vi "Main.vi"() -> ()   [LabVIEW 2020]
uses:
  <vilib>/MediaMongrels Ltd/WebSockets/Sockets/VISA TCP Listener/VISA TCP Listener.lvclass
  <vilib>/MediaMongrels Ltd/WebSockets/WebSockets/WebSocket Server/WebSocket Server.lvclass
  <vilib>/MediaMongrels Ltd/WebSockets/Sockets/Socket/Socket.lvclass
  <vilib>/Skyline/Tag/Wrapper/Wrapper_class/NI Skyline Tag.lvclass
  <vilib>/Skyline/Message/HTTP Wrapper/NI Skyline Message HTTP.lvclass
  <vilib>/Skyline/Tag/Shared/typedefs/DataType.ctl
  <vilib>/Skyline/Configuration/Configuration HTTP_class/NI Skyline Configuration HTTP.lvclass/NI Skyline Configuration HTTP.ctl
  <vilib>/Skyline/Configuration/Configuration HTTP_class/Open Configuration API Key.vi
  <vilib>/Skyline/Configuration/HTTP/Open Configuration API Key (Desktop).vi
  <vilib>/Skyline/Message/HTTP Wrapper/Open (HTTP).vi
  <vilib>/Skyline/Tag/Wrapper/Wrapper HTTP_class/Open Tag HTTP.vi
  <vilib>/Skyline/Tag/Wrapper/Wrapper_class/Write Tag (String).vi
  <vilib>/Skyline/Tag/Wrapper/Wrapper_class/Write Tag (Boolean).vi
  <vilib>/Skyline/Tag/Wrapper/Wrapper_class/Close Tag (Single).vi
  <vilib>/ErrorRing/Error Ring.xnode
  <vilib>/Skyline/Configuration/Configuration HTTP_class/NI Skyline Configuration HTTP.lvclass
  <vilib>/addons/_JKI.lib/Serialization/JSON/JKI JSON Serialization.lvlib
  <vilib>/Skyline/Configuration/Configuration_class/NI Skyline Configuration.lvclass
  <vilib>/Skyline/Tag/Shared/NI Skyline Tag.lvlib
  <vilib>/Skyline/Tag/Wrapper/Wrapper HTTP_class/NI Skyline Tag HTTP.lvclass
  <vilib>/Skyline/Message/NI Skyline Message.lvclass
panel:
  in  "Send SystemLink Messages?":bool
  in  "Send SystemLink Tags?":bool
  in  "Sync":bool
  out "Pi OS Time":string
  out "LV OS Time":string
  in  "LV Enabled":bool
  in  "LV OS Enabled":bool
  in  "Pi OS Enabled":bool
  in  "Pi OS TZ Update":bool
  in  "LV OS TZ Update":bool
  in  "LV TZ Update":bool
  out "LV Time":string
  in  "Timezone":string(combo)
  in  "Stop":bool
  # "Raspberry Pi WebSocket Server Example"
  # "This simple example sends the current date/time to the connected WebSocket Client.\n\nTo be used in conjunction with the corresponding NXG WebVI."
  # "Timezone\nUpdate"
  # "Update\nEnabled"
  # "Last Time Received"
  # "LabVIEW"
  # "LabVIEW OS"
  # "Pi OS"
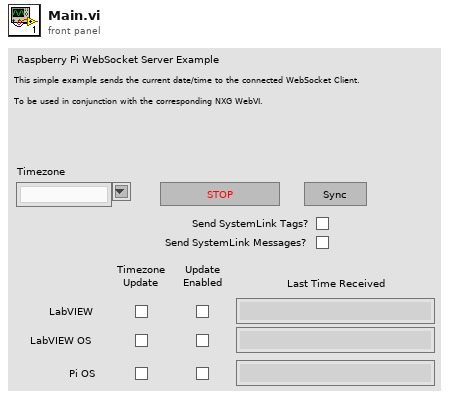
[diagram p1: front panel]
types:
  T1 = cluster{"Command":string, "Controls":cluster{"Name":string, "Value":bool}[]}
  T2 = typedef "NI Skyline Tag.lvlib/DataType.ctl" = enum32{"Double", "I32", "String", "Boolean", "U64", "Timestamp"}
  T3 = cluster{"Name":string, "Reference":refnum<class "NI Skyline Tag.lvclass">}
  T4 = cluster{"Core":cluster{"Current VI Reference":refnum<vi>}, "TCP Listener":refnum<class "VISA TCP Listener.lvclass">, "Socket":refnum<class "Socket.lvclass">, "WebSocket":refnum<class "WebSocket Server.lvclass">, "TCP Connection Info":cluster{"TCP Listen Port":u16, "Timeout (ms)":i32}, "Current Timezone":string, "Websocket Connected?":bool, "Current Time":cluster{"LabVIEW":string, "LabVIEW OS":string, "Pi OS":string}, "JSON Data In":string, "JSON Data Out":string, "Enabled Booleans":cluster{"LV Enabled":bool, "LV OS Enabled":bool, "Pi OS Enabled":bool}, "Timezone Booleans":cluster{"LV TZ Update":bool, "LV OS TZ Update":bool, "Pi OS TZ Update":bool}, "Initialized?":bool, "SystemLink Tag Info":cluster{"Name":string, "Reference":refnum<class "NI Skyline Tag.lvclass">}[], "SystemLink Booleans":cluster{"Send SystemLink Tags?":bool, "Send SystemLink Messages?":bool}, "SystemLink Message Session":refnum<class "NI Skyline Message HTTP.lvclass">}
  T5 = cluster{"Send SystemLink Tags?":bool, "Send SystemLink Messages?":bool}
  T6 = cluster{"Name":string, "Reference":refnum<class "NI Skyline Tag.lvclass">}[]
  T7 = cluster{"LV TZ Update":bool, "LV OS TZ Update":bool, "Pi OS TZ Update":bool}
  T8 = cluster{"LV Enabled":bool, "LV OS Enabled":bool, "Pi OS Enabled":bool}
  T9 = cluster{"LabVIEW":string, "LabVIEW OS":string, "Pi OS":string}
  T10 = cluster{"TCP Listen Port":u16, "Timeout (ms)":i32}
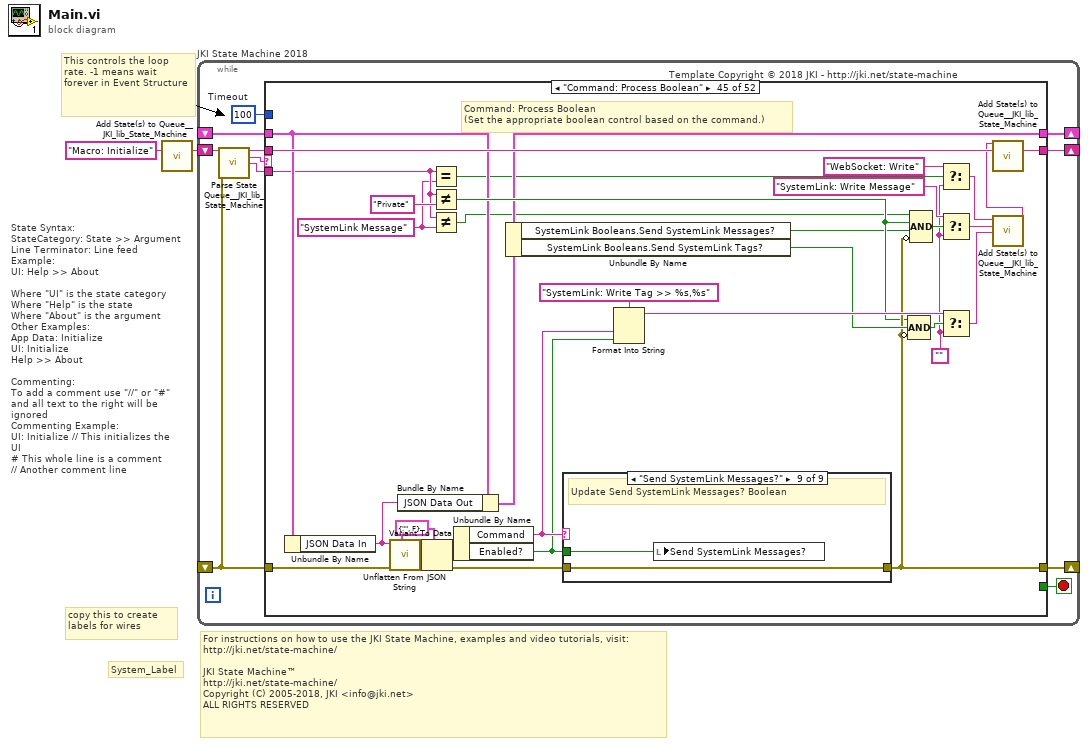
[diagram p0: block diagram]
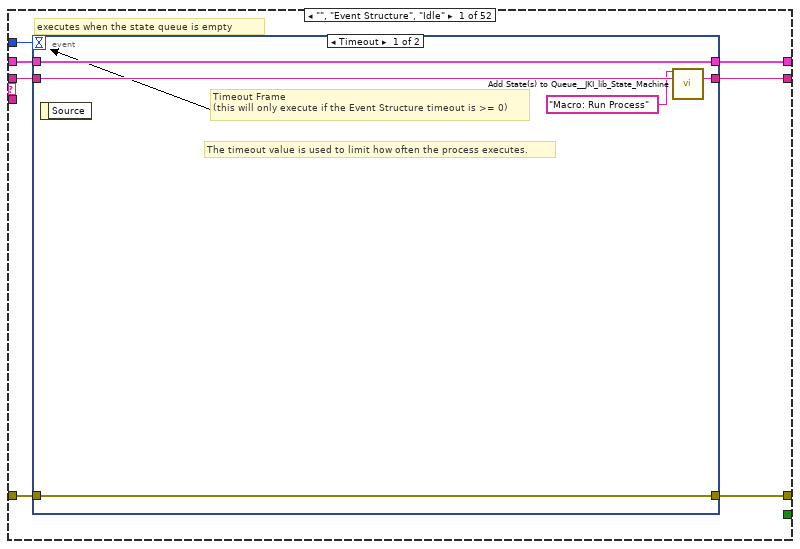
[diagram p2: hidden frame]
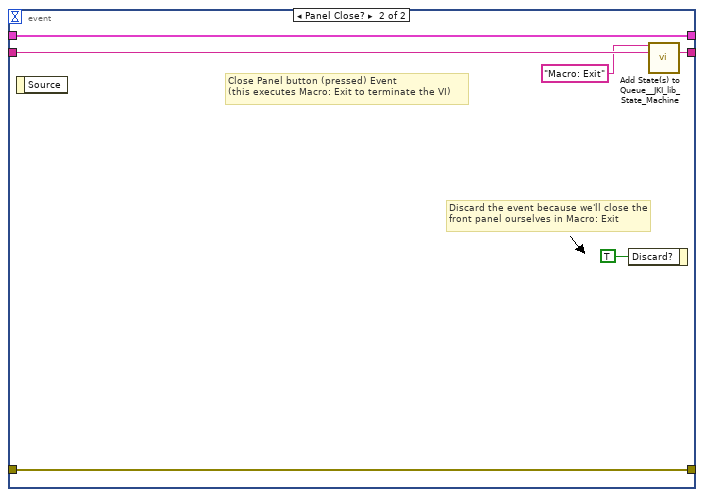
[diagram p3: hidden frame]
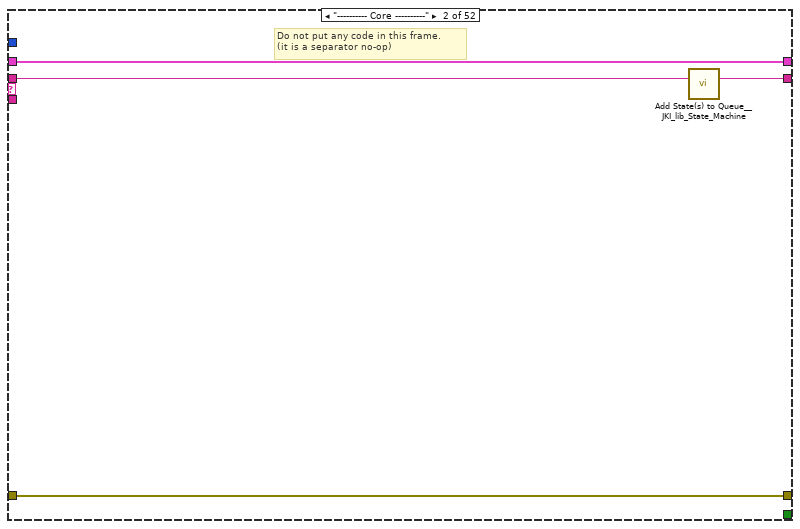
[diagram p4: hidden frame]
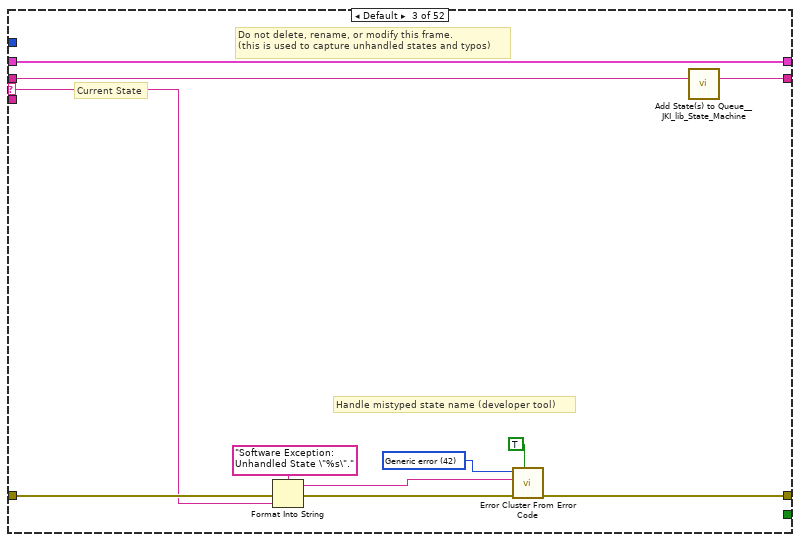
[diagram p5: hidden frame]
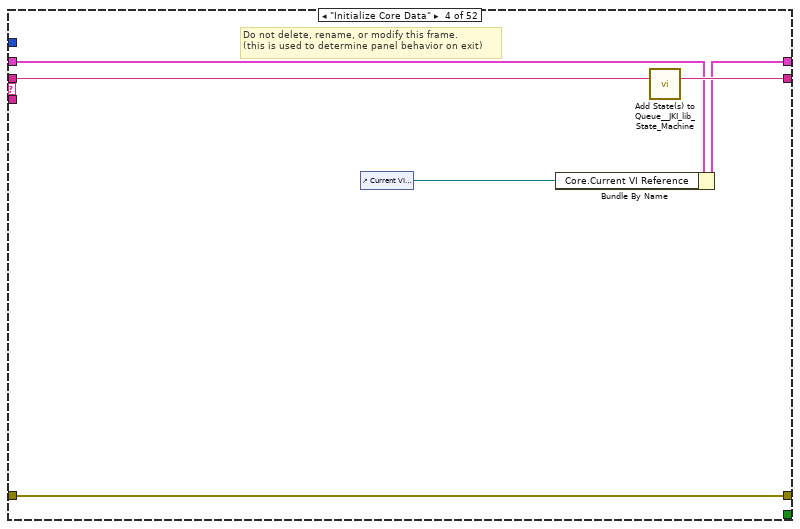
[diagram p6: hidden frame]
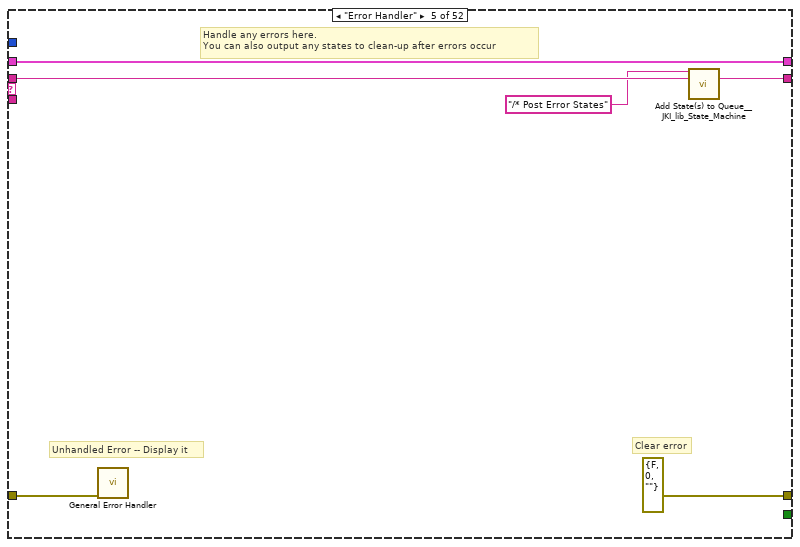
[diagram p7: hidden frame]
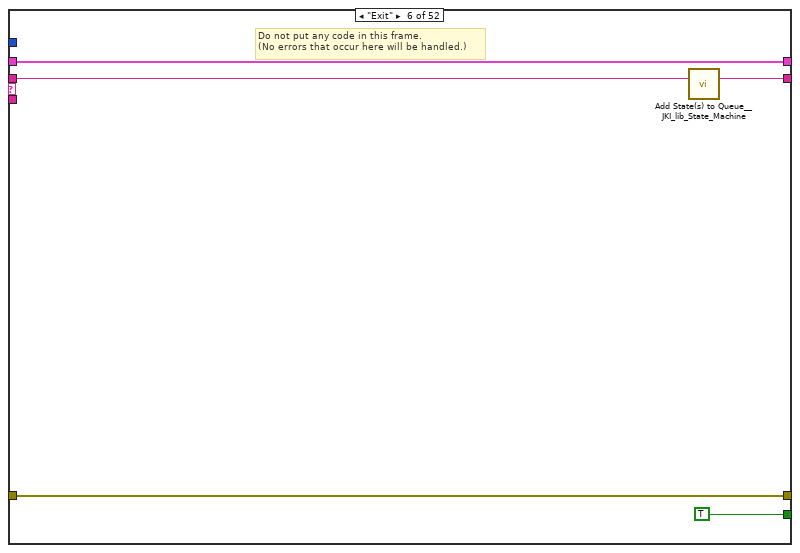
[diagram p8: hidden frame]
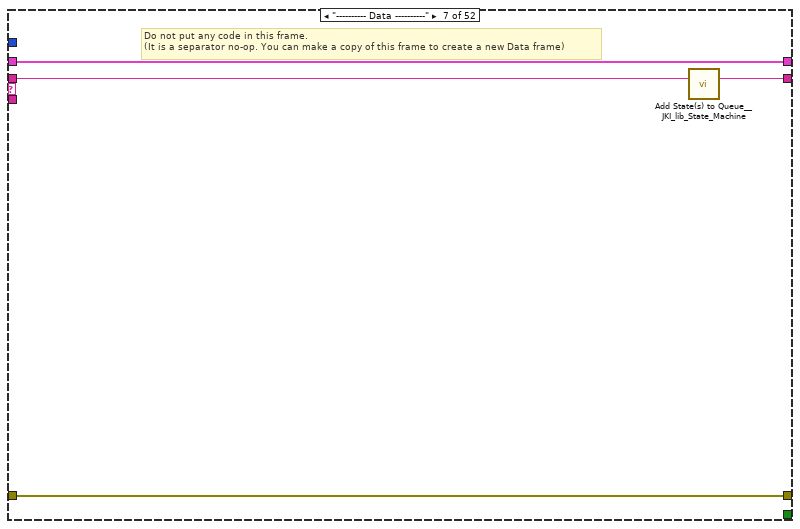
[diagram p9: hidden frame]
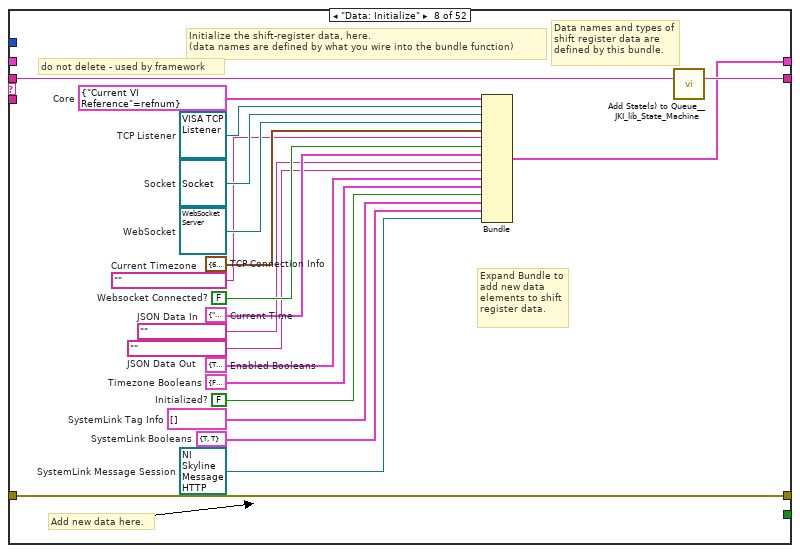
[diagram p10: hidden frame]
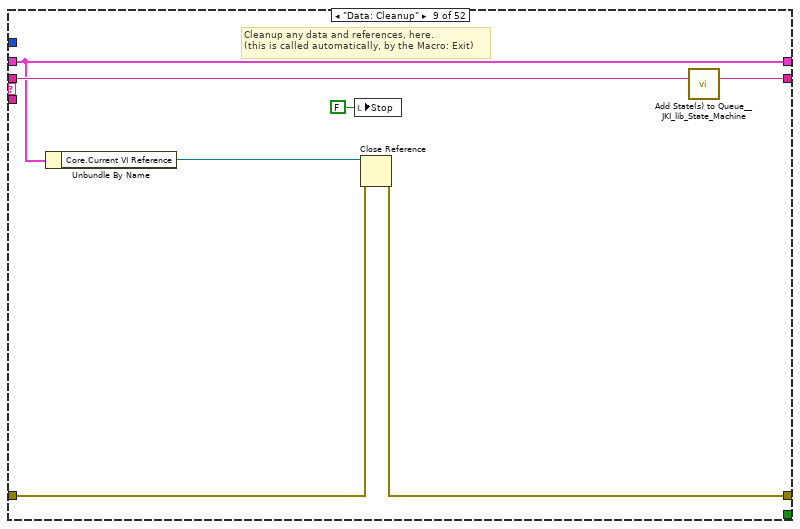
[diagram p11: hidden frame]
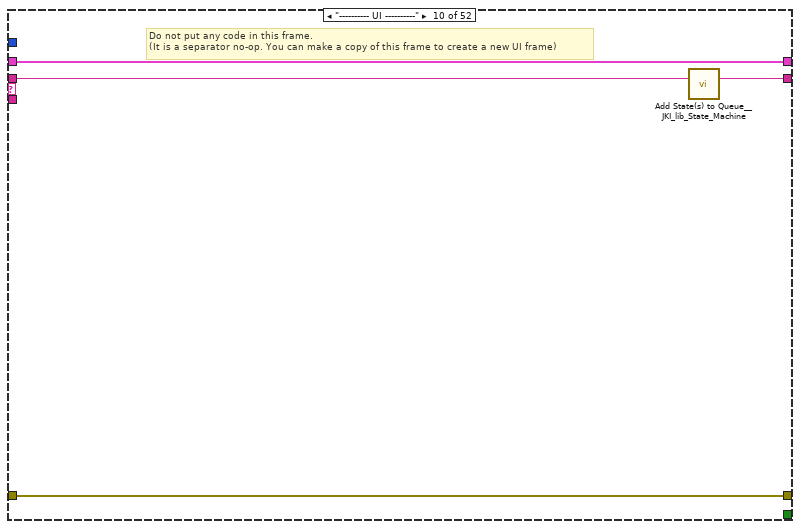
[diagram p12: hidden frame]
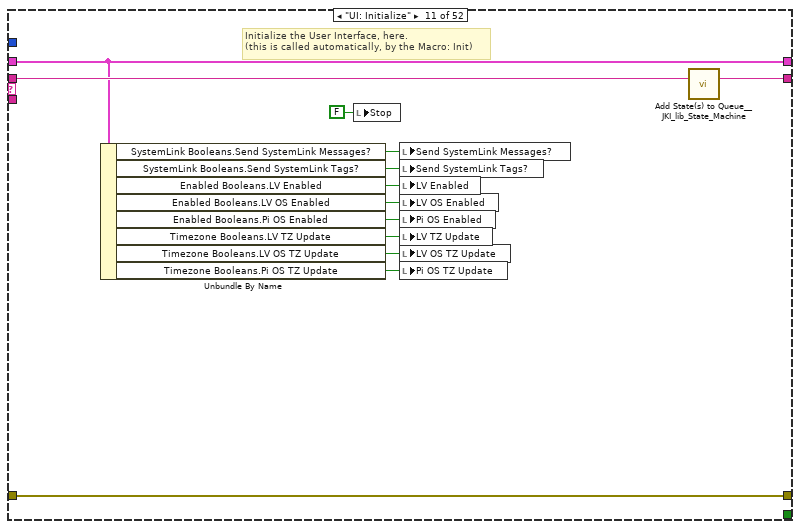
[diagram p13: hidden frame]
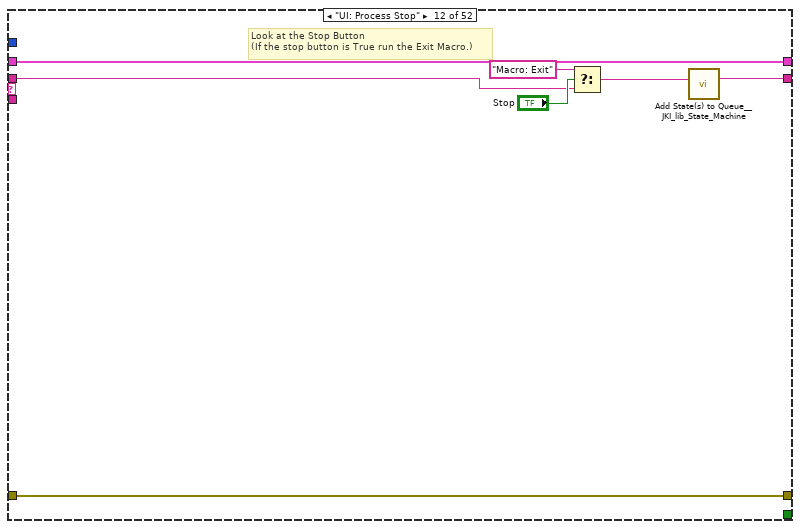
[diagram p14: hidden frame]
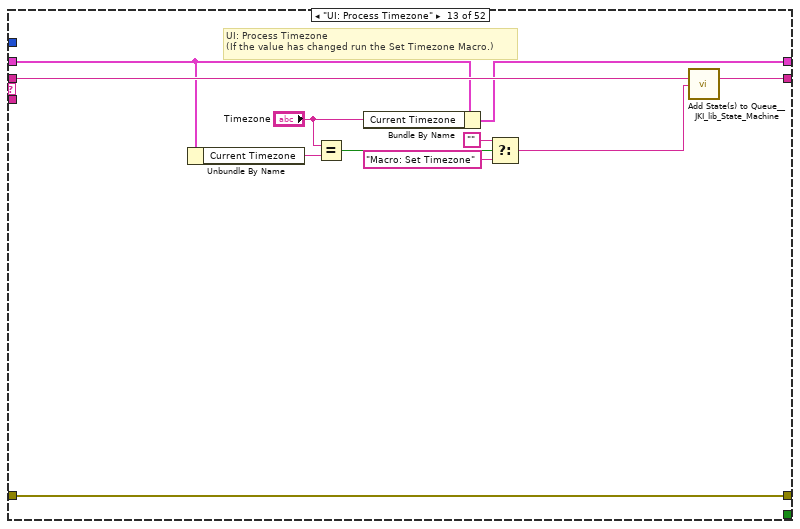
[diagram p15: hidden frame]
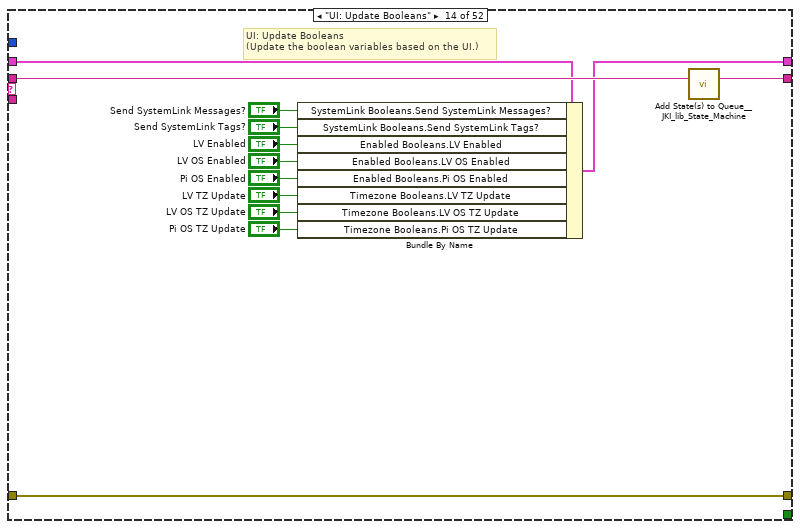
[diagram p16: hidden frame]
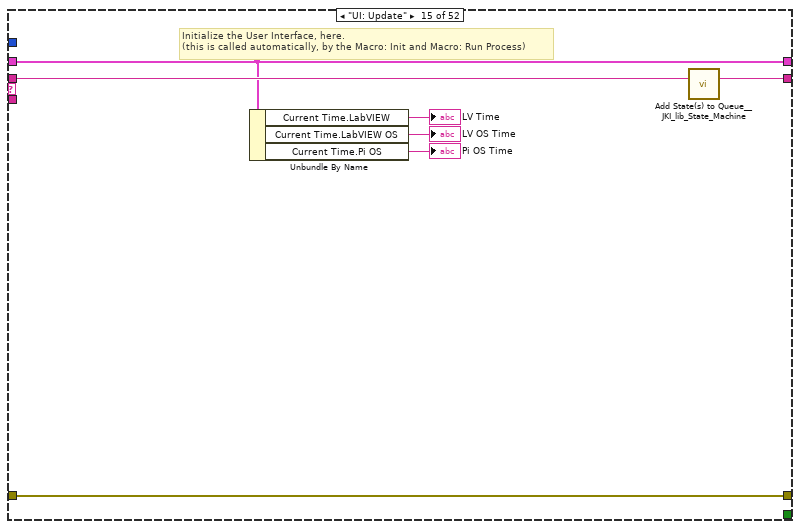
[diagram p17: hidden frame]
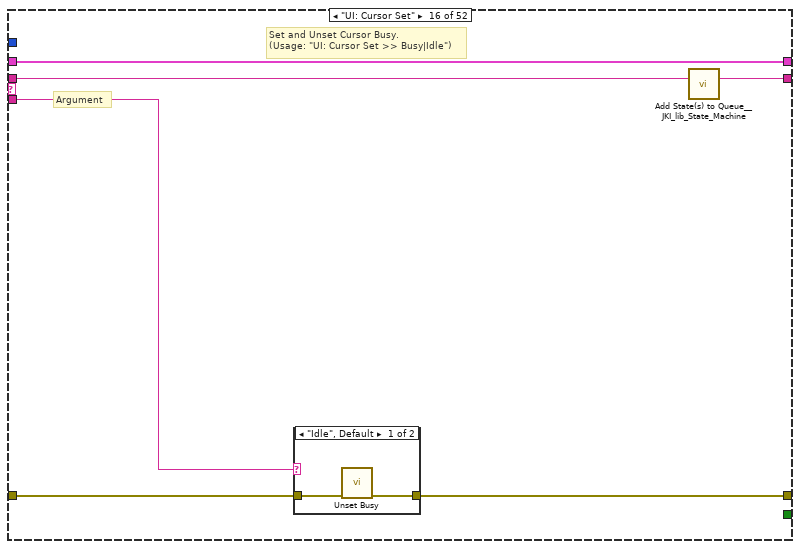
[diagram p18: hidden frame]
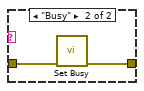
[diagram p19: hidden frame]
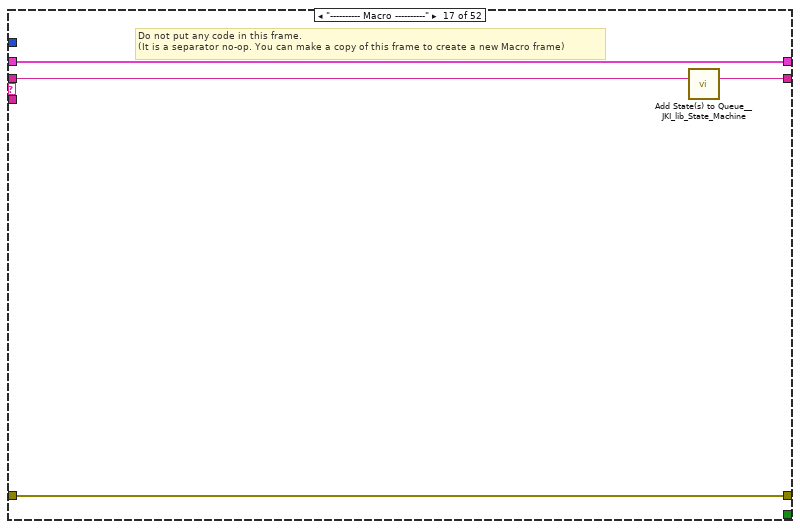
[diagram p20: hidden frame]
diagram:
  # "For instructions on how to use the JKI State Machine, examples and video tutorials, visit:\nhttp://jki.net/state-machine/\n\nJKI State Machine™\nhttp://jki.net/state-machine/\nCopyright (C) 2005-2018, JKI <info@jki.net>\nALL RIGHTS RESERVED"
  # "State Syntax:\nStateCategory: State >> Argument\nLine Terminator: Line feed\nExample:\nUI: Help >> About\n\nWhere \"UI\" is the state category\nWhere \"Help\" is the state\nWhere \"About\" is the argument\nOther Examples:\nApp Data: Initialize\nUI: Initialize\nHelp >> About\n\nCommenting:\nTo add a comment use \"//\" or \"#\" and all text to the right will be ignored\nCommenting Example:\nUI: Initialize // This initializes the UI\n# This whole line is a comment\n// Another comment line"
  # "copy this to create labels for wires"
  # "This controls the loop rate. -1 means wait forever in Event Structure"
  # "System_Label"
  n1 = call <vilib>:"Add State(s) to Queue__JKI_lib_State_Machine.vi"("State(s) in (\"\")"="Macro: Initialize") -> ("States Out"=w2:string)  [unwired: 14 in]
  n2 = while "JKI State Machine 2018" {
    shift-right: [w6] -> _
    shift-left: _ -> [w5]
    shift-right: [w9] -> _
    shift-left: _ -> [w3]
    shift-right: [w8] -> _
    shift-left: w2 -> [w10]
    stop <- w7 stop-if-true
    w4 = 100  # Timeout
    # "Template Copyright © 2018 JKI - http://jki.net/state-machine"
    n3 = call <vilib>:"Parse State Queue__JKI_lib_State_Machine.vi"("State Queue"=w10, "Error In (no error)"=w3) -> ("Remaining States"=w12:string, "Current State"=w13:string, "Arguments"=w11:string)  [unwired: 11 in]
    n4 = case shown="\"Command: Process Boolean\"" w13 {
      selector: w13 -> [_ _ w36 _ _ _ _ _ _ _ _ _ _ _ _ _ _ _ _ _ _ _ _ _ _ _ _ _ _ _ _ _ _ _ _ _ _ _ _ _ _ _ _ _ _ _ _ _ _ _ _ _]
      tunnel: w12 -> [w20 w35 w40 w52 w58 w63 w67 w87 w94 w98 w111 w114 w127 w141 w149 w155 w163 w168 w194 w212 w217 w221 w242 w256 w273 w280 w295 w319 w341 w343 w365 w381 w397 w405 w413 w419 w423 w437 w446 w482 w514 w532 w548 w565 w598 w636 w670 w688 w710 w730 w789 w796]
      tunnel: w11 -> [_ _ _ _ _ _ _ _ _ _ _ _ _ _ _ w150 _ _ _ _ _ _ _ _ w264 _ _ _ _ w345 _ _ _ _ _ _ _ _ _ _ w500 w516 _ _ w571 _ _ _ _ w726 _ _]
      tunnel: w5 -> [w18 w32 w38 w48 w55 w61 w64 _ w89 w95 w107 w116 w121 w140 w146 w153 w160 w165 w191 w199 w214 w218 w232 w248 w269 w277 w289 w312 w338 w350 w362 w367 w383 w401 w407 w417 w420 w425 w440 w463 w499 w522 w545 w553 w575 w628 w667 w684 w708 w715 w783 w791]
      tunnel: [w17 w33 w42 w49 errorcluster {"status"=FALSE, "code"=0, "source"=""} ("error out") w60 w65 w85 w90 w96 w109 w117 w128 w138 w147 w151 w161 w166 w192 w210 w215 w219 w226 w250 w265 w278 w287 w311 w330 w346 w363 w371 w387 w398 w408 w415 w421 w428 w441 w479 w512 w523 w546 w560 w582 w625 w668 w682 w704 w727 w784 w792] -> w9
      tunnel: w3 -> [w16 w33 w41 w49 w54 w60 w65 w85 w91 w96 w109 w117 w128 w138 w147 w152 w161 w166 w192 w210 w215 w219 w238 w253 w271 w278 w291 w316 w333 w352 w363 w375 w392 w399 w409 w416 w421 w429 w442 w480 w512 w524 w546 w559 w595 w633 w668 w681 w707 w728 w785 w794]
      tunnel: [w19 w34 w39 w51 w57 w62 w66 w86 w93 w97 w110 w118 w129 w142 w148 w154 w162 w167 w193 w211 w216 w220 w241 w255 w272 w279 w294 w318 w340 w354 w364 w380 w396 w404 w412 w418 w422 w436 w445 w481 w513 w531 w547 w564 w597 w635 w669 w687 w709 w729 w788 w795] -> w8
      tunnel: [_ _ _ _ _ TRUE _ _ _ _ _ _ _ _ _ _ _ _ _ _ _ _ _ _ _ _ _ _ _ _ _ _ _ _ _ _ _ _ _ _ _ _ _ _ _ _ _ _ _ _ _ _] -> w7
      tunnel: [w15 w32 w38 w50 w55 w61 w64 w71 w89 w95 w107 w116 w120 w139 w146 w153 w160 w165 w191 w199 w214 w218 w230 w252 w267 w277 w284 w309 w337 w348 w362 w376 w391 w401 w407 w417 w420 w435 w438 w477 w499 w522 w545 w552 w573 w628 w667 w683 w702 w714 w781 w791] -> w6
      tunnel: w4 -> [w14 _ _ _ _ _ _ _ _ _ _ _ _ _ _ _ _ _ _ _ _ _ _ _ _ _ _ _ _ _ _ _ _ _ _ _ _ _ _ _ _ _ _ _ _ _ _ _ _ _ _ _]
      frame "", "Event Structure", "Idle" {
        # "executes when the state queue is empty"
        n5 = event shown="[0] Timeout" {
          selector: _ -> [_ _]
          dyn-events: _ -> [_ _]
          timeout: w14 -> [_ _]
          tunnel: w20 -> [w25 w31]
          tunnel: [w24 w30] -> w19
          tunnel: w18 -> [w22 w28]
          tunnel: [w23 w29] -> w17
          tunnel: w16 -> [w23 w29]
          tunnel: [w22 w28] -> w15
          event Timeout {
            # "The timeout value is used to limit how often the process executes."
            # "Timeout Frame\n(this will only execute if the Event Structure timeout is >= 0)"
            n6 = event-data() -> ()  [unwired: 1 in, 1 out]
            n7 = call <vilib>:"Add State(s) to Queue__JKI_lib_State_Machine.vi"("State(s) in Front (\"\")"="Macro: Run Process", "State(s) in (\"\")"=w25) -> ("States Out"=w24:string)  [unwired: 13 in]
          }
          event Panel Close? {
            # "Discard the event because we'll close the front panel ourselves in Macro: Exit"
            # "Close Panel button (pressed) Event\n(this executes Macro: Exit to terminate the VI)"
            n8 = event-data() -> ()  [unwired: 1 in, 1 out]
            n9 = event-data("Discard?"=TRUE) -> ()  [unwired: 1 in, 1 out]
            n10 = call <vilib>:"Add State(s) to Queue__JKI_lib_State_Machine.vi"("State(s) in Front (\"\")"="Macro: Exit", "State(s) in (\"\")"=w31) -> ("States Out"=w30:string)  [unwired: 13 in]
          }
        }
      }
      frame "---------- Core ----------" {
        # "Do not put any code in this frame.\n(it is a separator no-op)"
        n11 = call <vilib>:"Add State(s) to Queue__JKI_lib_State_Machine.vi"("State(s) in (\"\")"=w35) -> ("States Out"=w34:string)  [unwired: 14 in]
      }
      frame Default {
        w45 = 42 items=["No error", "Argument error", "Memory is full", "Out of zone", "End of file", "File already open", "Generic file I/O error", "File not found", "File permission error", "Disk is full", "Duplicate path", "Too many files open", "System feature not enabled", "Resource file not found", "Cannot add resource", "Resource not found", "Image not found", "Image memory error", "Pen does not exist", "Config type invalid", "Config token not found", "Config parse error", "Config memory error", "Bad external code format", "Bad external code offset", "External code not present", "Null window", "Destroy window error", "Null menu", "Print aborted", "Bad print record", "Print driver error", "Windows error during printing", "Memory error during printing", "Print dialog error", "Generic print error", "Invalid device refnum", "Device not found", "Device parameter error", "Device unit error", "Cannot open device", "Device call aborted", "Generic error", "Cancelled by user", "Object ID too low", "Object ID too high", "Object not in heap", "Unknown heap", "Unknown object (invalid DefProc)", "Unknown object (DefProc not in table)", "Message out of range", "Invalid (null) method", "Unknown message", "Manager call not supported", "Bad address", "Network operation in progress", "Network operation timed out", "Connection is busy", "Network attribute not supported", "Network error", "Address in use", "System out of memory", "Connection aborted", "Connection refused", "Not connected", "Already connected", "Connection closed", "Initialization error (interapplication manager)", "Bad occurrence", "Wait on unbound occurrence handler", "Occurrence queue overflow", "Datalog type conflict", "Unused", "Unrecognized type (interapplication manager)", "Memory corrupt", "Failed to make temporary DLL", "Old CIN version", "Drag socket not found", "Failed to load drop-object", "Failed to register OLE object", "Failed to release OLE object", "Format specifier type mismatch", "Unknown format specifier", "Too few format specifiers", "Too many format specifiers", "Scan failed", "Newer CIN version", "Error converting to variant", "Runtime menu error", "Password tampered", "Variant attribute not found", "Incompatible variant data type", "Event data is not available", "Event Store is not present", "Occurrence is not found", "Event Queue is not created", "Event info is not available", "Refnum passed is NULL", "Error retrieving Class GUID", "Error retrieving CoClass GUID", "Error retrieving TypeLib GUID.", "Bad built application magic bytes.", "Specific driver is different from the specific driver associated with the Logical Name.", "There is no session opened to the class driver.", "Max Error", "MAX - Error with config objects", "MAX - Error loading configuration", "MAX - Group not supported"]
        # "Current State"
        # "Do not delete, rename, or modify this frame.\n(this is used to capture unhandled states and typos)"
        # "Handle mistyped state name (developer tool)"
        n12 = Format Into String(format string="Software Exception: Unhandled State \"%s\"." ("message"), error in=w41, w36) -> (resulting string=w44:string, error out=w43:errorcluster)  [unwired: 1 in]
        n13 = call <vilib>:"Error Cluster From Error Code.vi"("show call chain? (False)"=TRUE, "error in (no error)"=w43, "error message (\"\")"=w44, "error code (0)"=w45) -> ("error out"=w42:errorcluster)  [unwired: 5 in]
        n14 = call <vilib>:"Add State(s) to Queue__JKI_lib_State_Machine.vi"("State(s) in (\"\")"=w40) -> ("States Out"=w39:string)  [unwired: 14 in]
      }
      frame "Initialize Core Data" {
        # "Do not delete, rename, or modify this frame.\n(this is used to determine panel behavior on exit)"
        n15 = control-ref of="Current VI Reference"() -> (w47:refnum<vi>)
        n16 = Bundle By Name(cluster=w48, "Core.Current VI Reference"=w47) -> (w50:T4)
        n17 = call <vilib>:"Add State(s) to Queue__JKI_lib_State_Machine.vi"("State(s) in (\"\")"=w52) -> ("States Out"=w51:string)  [unwired: 14 in]
      }
      frame "Error Handler" {
        # "Unhandled Error -- Display it"
        # "Handle any errors here.\nYou can also output any states to clean-up after errors occur"
        # "Clear error"
        n18 = call <vilib>:"General Error Handler.vi"("error in (no error)"=w54) -> ()  [unwired: 10 in, 5 out]
        n19 = call <vilib>:"Add State(s) to Queue__JKI_lib_State_Machine.vi"("State(s) in Front (\"\")"="/* Post Error States", "State(s) in (\"\")"=w58) -> ("States Out"=w57:string)  [unwired: 13 in]
      }
      frame "Exit" {
        # "Do not put any code in this frame.\n(No errors that occur here will be handled.)"
        n20 = call <vilib>:"Add State(s) to Queue__JKI_lib_State_Machine.vi"("State(s) in (\"\")"=w63) -> ("States Out"=w62:string)  [unwired: 14 in]
      }
      frame "---------- Data ----------" {
        # "Do not put any code in this frame.\n(It is a separator no-op. You can make a copy of this frame to create a new Data frame)"
        n21 = call <vilib>:"Add State(s) to Queue__JKI_lib_State_Machine.vi"("State(s) in (\"\")"=w67) -> ("States Out"=w66:string)  [unwired: 14 in]
      }
      frame "Data: Initialize" {
        w68 = T5 {"Send SystemLink Tags?"=TRUE, "Send SystemLink Messages?"=TRUE}  # SystemLink Booleans
        w69 = refnum<class "NI Skyline Message HTTP.lvclass"> refnum  # SystemLink Message Session
        w70 = T6 []  # SystemLink Tag Info
        w72 = FALSE  # Initialized?
        w73 = T7 {"LV TZ Update"=FALSE, "LV OS TZ Update"=TRUE, "Pi OS TZ Update"=TRUE}  # Timezone Booleans
        w74 = T8 {"LV Enabled"=TRUE, "LV OS Enabled"=TRUE, "Pi OS Enabled"=TRUE}  # Enabled Booleans
        w75 = ""  # JSON Data Out
        w76 = ""  # JSON Data In
        w77 = T9 {"LabVIEW"="", "LabVIEW OS"="", "Pi OS"=""}  # Current Time
        w78 = FALSE  # Websocket Connected?
        w79 = ""  # Current Timezone
        w80 = refnum<class "Socket.lvclass"> refnum  # Socket
        w82 = T10 {"TCP Listen Port"=6123, "Timeout (ms)"=1000}  # TCP Connection Info
        w81 = refnum<class "WebSocket Server.lvclass"> refnum  # WebSocket
        w83 = refnum<class "VISA TCP Listener.lvclass"> refnum  # TCP Listener
        w84 = cluster{"Current VI Reference":refnum<vi>} {"Current VI Reference"=refnum}  # Core
        # "do not delete - used by framework"
        # "Expand Bundle to add new data elements to shift register data."
        # "Add new data here."
        # "Data names and types of shift register data are defined by this bundle."
        # "Initialize the shift-register data, here.\n(data names are defined by what you wire into the bundle function)"
        n22 = Bundle("Core"=w84, "TCP Listener"=w83, "Socket"=w80, "WebSocket"=w81, "TCP Connection Info"=w82, "Current Timezone"=w79, "Websocket Connected?"=w78, "Current Time"=w77, "JSON Data In"=w76, "JSON Data Out"=w75, "Enabled Booleans"=w74, "Timezone Booleans"=w73, "Initialized?"=w72, "SystemLink Tag Info"=w70, "SystemLink Booleans"=w68, "SystemLink Message Session"=w69) -> (w71:T4)  [unwired: 1 in]
        n23 = call <vilib>:"Add State(s) to Queue__JKI_lib_State_Machine.vi"("State(s) in (\"\")"=w87) -> ("States Out"=w86:string)  [unwired: 14 in]
      }
      frame "Data: Cleanup" {
        # "Cleanup any data and references, here.\n(this is called automatically, by the Macro: Exit)"
        n24 = Unbundle By Name(w89) -> ("Core.Current VI Reference"=w92:refnum<vi>)
        n25 = local write "Stop"(FALSE ("Stop")) -> ()
        n26 = Close Reference(reference=w92, error in (no error)=w91) -> (error out=w90:errorcluster)
        n27 = call <vilib>:"Add State(s) to Queue__JKI_lib_State_Machine.vi"("State(s) in (\"\")"=w94) -> ("States Out"=w93:string)  [unwired: 14 in]
      }
      frame "---------- UI ----------" {
        # "Do not put any code in this frame.\n(It is a separator no-op. You can make a copy of this frame to create a new UI frame)"
        n28 = call <vilib>:"Add State(s) to Queue__JKI_lib_State_Machine.vi"("State(s) in (\"\")"=w98) -> ("States Out"=w97:string)  [unwired: 14 in]
      }
      frame "UI: Initialize" {
        # "Initialize the User Interface, here.\n(this is called automatically, by the Macro: Init)"
        n29 = Unbundle By Name(w107) -> ("SystemLink Booleans.Send SystemLink Messages?"=w99:bool, "SystemLink Booleans.Send SystemLink Tags?"=w100:bool, "Enabled Booleans.LV Enabled"=w106:bool, "Enabled Booleans.LV OS Enabled"=w105:bool, "Enabled Booleans.Pi OS Enabled"=w104:bool, "Timezone Booleans.LV TZ Update"=w103:bool, "Timezone Booleans.LV OS TZ Update"=w102:bool, "Timezone Booleans.Pi OS TZ Update"=w101:bool)
        n30 = local write "Stop"(FALSE ("Stop")) -> ()
        n31 = local write "Send SystemLink Messages?"(w99) -> ()
        n32 = local write "Send SystemLink Tags?"(w100) -> ()
        n33 = local write "LV Enabled"(w106) -> ()
        n34 = local write "LV OS Enabled"(w105) -> ()
        n35 = local write "Pi OS Enabled"(w104) -> ()
        n36 = local write "LV TZ Update"(w103) -> ()
        n37 = local write "LV OS TZ Update"(w102) -> ()
        n38 = local write "Pi OS TZ Update"(w101) -> ()
        n39 = call <vilib>:"Add State(s) to Queue__JKI_lib_State_Machine.vi"("State(s) in (\"\")"=w111) -> ("States Out"=w110:string)  [unwired: 14 in]
      }
      frame "UI: Process Stop" {
        # "Look at the Stop Button\n(If the stop button is True run the Exit Macro.)"
        n40 = Select(t="Macro: Exit", s="Stop", f=w114) -> (s? t:f=w113:string)
        n41 = call <vilib>:"Add State(s) to Queue__JKI_lib_State_Machine.vi"("State(s) in (\"\")"=w113) -> ("States Out"=w118:string)  [unwired: 14 in]
      }
      frame "UI: Process Timezone" {
        # "UI: Process Timezone\n(If the value has changed run the Set Timezone Macro.)"
        n42 = Unbundle By Name(w121) -> ("Current Timezone"=w122:string)
        n43 = Equal?(x="Timezone", y=w122) -> (x = y?=w126:bool)
        n44 = Bundle By Name(cluster=w121, "Current Timezone"="Timezone") -> (w120:T4)
        n45 = Select(t="", s=w126, f="Macro: Set Timezone") -> (s? t:f=w124:string)
        n46 = call <vilib>:"Add State(s) to Queue__JKI_lib_State_Machine.vi"("State(s) in (\"\")"=w127, "State(s) at Back (\"\")"=w124) -> ("States Out"=w129:string)  [unwired: 13 in]
      }
      frame "UI: Update Booleans" {
        # "UI: Update Booleans\n(Update the boolean variables based on the UI.)"
        n47 = Bundle By Name(cluster=w140, "SystemLink Booleans.Send SystemLink Messages?"="Send SystemLink Messages?", "SystemLink Booleans.Send SystemLink Tags?"="Send SystemLink Tags?", "Enabled Booleans.LV Enabled"="LV Enabled", "Enabled Booleans.LV OS Enabled"="LV OS Enabled", "Enabled Booleans.Pi OS Enabled"="Pi OS Enabled", "Timezone Booleans.LV TZ Update"="LV TZ Update", "Timezone Booleans.LV OS TZ Update"="LV OS TZ Update", "Timezone Booleans.Pi OS TZ Update"="Pi OS TZ Update") -> (w139:T4)
        n48 = call <vilib>:"Add State(s) to Queue__JKI_lib_State_Machine.vi"("State(s) in (\"\")"=w141) -> ("States Out"=w142:string)  [unwired: 14 in]
      }
      frame "UI: Update" {
        # "Initialize the User Interface, here.\n(this is called automatically, by the Macro: Init and Macro: Run Process)"
        n49 = Unbundle By Name(w146) -> ("Current Time.LabVIEW"=→"LV Time":string, "Current Time.LabVIEW OS"=→"LV OS Time":string, "Current Time.Pi OS"=→"Pi OS Time":string)
        n50 = call <vilib>:"Add State(s) to Queue__JKI_lib_State_Machine.vi"("State(s) in (\"\")"=w149) -> ("States Out"=w148:string)  [unwired: 14 in]
      }
      frame "UI: Cursor Set" {
        # "Argument"
        # "Set and Unset Cursor Busy.\n(Usage: \"UI: Cursor Set >> Busy|Idle\")"
        n51 = case shown="\"Idle\", Default" w150 {
          tunnel: w152 -> [w157 w159]
          tunnel: [w156 w158] -> w151
          frame "Idle", Default {
            n52 = call <vilib>:"Unset Busy.vi"("error in (no error)"=w157) -> ("error out"=w156:errorcluster)  [unwired: 10 in]
          }
          frame "Busy" {
            n53 = call <vilib>:"Set Busy.vi"("error in (no error)"=w159) -> ("error out"=w158:errorcluster)  [unwired: 9 in, 1 out]
          }
        }
        n54 = call <vilib>:"Add State(s) to Queue__JKI_lib_State_Machine.vi"("State(s) in (\"\")"=w155) -> ("States Out"=w154:string)  [unwired: 14 in]
      }
      frame "---------- Macro ----------" {
        # "Do not put any code in this frame.\n(It is a separator no-op. You can make a copy of this frame to create a new Macro frame)"
        n55 = call <vilib>:"Add State(s) to Queue__JKI_lib_State_Machine.vi"("State(s) in (\"\")"=w163) -> ("States Out"=w162:string)  [unwired: 14 in]
      }
      frame "Macro: Initialize" {
        # "Initialization Macro\n(This is called once, when the VI starts)"
        n56 = call <vilib>:"Add State(s) to Queue__JKI_lib_State_Machine.vi"("State(s) in Front (\"\")"="Data: Initialize\nInitialize Core Data\nUI: Initialize\nSystemLink: Initialize\nTCP: Initialize", "State(s) in (\"\")"=w168) -> ("States Out"=w167:string)  [unwired: 13 in]
      }
      frame "Macro: Run Process" {
        # "Process Macro\n(Put everything in here that runs in a loop when connected.)"
        n57 = Unbundle By Name(w191) -> ("Enabled Booleans.LV Enabled"=w184:bool, "Enabled Booleans.LV OS Enabled"=w176:bool, "Enabled Booleans.Pi OS Enabled"=w173:bool, "Websocket Connected?"=w190:bool)
        n58 = Select(t="Project: Sync Web UI", s="Sync", f="") -> (s? t:f=w169:string)
        n59 = Select(t="Project: Get LabVIEW Time", s=w184, f="") -> (s? t:f=w178:string)
        n60 = Select(t="Pi: Get LabVIEW OS Time", s=w176, f="") -> (s? t:f=w177:string)
        n61 = Select(t="Pi: Get Pi OS Time", s=w173, f="") -> (s? t:f=w174:string)
        n62 = Select(t="WebSocket: Read", s=w190, f="") -> (s? t:f=w175:string)
        n63 = Format Into String(format string="UI: Process Stop\n%s\n%s\n%s\n%s\n%s\nSystemLink: Read Message\nUI: Process Timezone\nUI: Update Booleans\nUI: Update", w169, w178, w177, w174, w175) -> (resulting string=w183:string)  [unwired: 2 in, 1 out]
        n64 = call <vilib>:"Add State(s) to Queue__JKI_lib_State_Machine.vi"("State(s) in Front (\"\")"=w183, "State(s) in (\"\")"=w194) -> ("States Out"=w193:string)  [unwired: 13 in]
      }
      frame "Macro: Set Timezone" {
        # "Set Timezone Macro\n(Process the Timezone change. )"
        n65 = Unbundle By Name(w199) -> ("Timezone Booleans.LV OS TZ Update"=w201:bool, "Timezone Booleans.Pi OS TZ Update"=w200:bool, "Timezone Booleans.LV TZ Update"=w196:bool)
        n66 = Select(t="Pi: Set LabVIEW OS Timezone", s=w201, f="") -> (s? t:f=w204:string)
        n67 = Select(t="Pi: Set Pi OS Timezone", s=w200, f="") -> (s? t:f=w203:string)
        n68 = Select(t="Pi: Restart LabVIEW Service", s=w196, f="") -> (s? t:f=w195:string)
        n69 = Format Into String(format string="%s\n%s", w204, w203) -> (resulting string=w202:string)  [unwired: 2 in, 1 out]
        n70 = call <vilib>:"Add State(s) to Queue__JKI_lib_State_Machine.vi"("State(s) in Front (\"\")"=w202, "State(s) in (\"\")"=w212, "State(s) at Back (\"\")"=w195) -> ("States Out"=w211:string)  [unwired: 12 in]
      }
      frame "Macro: Exit" {
        # "On exit we don't know the current state of the program \nso try to close all connections and ignore errors."
        # "Exit Macro\n(This is called once, when the VI exits)"
        n71 = call <vilib>:"Add State(s) to Queue__JKI_lib_State_Machine.vi"("State(s) in Front (\"\")"="WebSocket: Close >> Ignore Errors\nTCP: Close >> Ignore Errors\nSystemLink: Close\nData: Cleanup\nExit", "State(s) in (\"\")"=w217) -> ("States Out"=w216:string)  [unwired: 13 in]
      }
      frame "---------- TCP ----------" {
        # "Do not put any code in this frame.\n(It is a separator no-op. You can make a copy of this frame to create a new TCP frame)"
        n72 = call <vilib>:"Add State(s) to Queue__JKI_lib_State_Machine.vi"("State(s) in (\"\")"=w221) -> ("States Out"=w220:string)  [unwired: 14 in]
      }
      frame "TCP: Initialize" {
        # "On Error repeat the initializion \nuntil a valid connection is made."
        # "TCP: Initialize\n(Close any open TCP connection and open a new connection.)"
        n73 = Unbundle By Name(w232) -> ("Initialized?"=w223:bool, "TCP Connection Info.TCP Listen Port"=w233:u16, "TCP Connection Info.Timeout (ms)"=w234:i32, "TCP Listener"=w237:refnum<class "VISA TCP Listener.lvclass">)
        n74 = call-dynamic "Close.vi"("error in (no error)"=w238, "VISA TCP Listener in"=w237) -> ("error out"=w240:errorcluster)  [unwired: 9 in]
        n75 = call <vilib>:"Clear Errors.vi"("error in (no error)"=w240) -> ("error out"=w239:errorcluster)  [unwired: 5 in, 1 out]
        n76 = call <vilib>:"New VISA TCP Listener.vi"("error in (no error)"=w239) -> ("error out"=w235:errorcluster, "VISA TCP Listener out"=w236:refnum<class "VISA TCP Listener.lvclass">)  [unwired: 9 in]
        n77 = call-dynamic "Create Listener.vi"("error in (no error)"=w235, "timeout ms (5000)"=w234, "Port"=w233, "VISA TCP Listener in"=w236) -> ("error out"=w224:errorcluster, "VISA TCP Listener out"=w231:refnum<class "VISA TCP Listener.lvclass">)  [unwired: 6 in]
        n78 = Select(t="Macro: Run Process\nTCP: Initialize", s=w224, f="TCP: Listen") -> (s? t:f=w228:string)
        n79 = Select(t=TRUE, s=w224, f=w223) -> (s? t:f=w225:bool)
        n80 = Bundle By Name(cluster=w232, "Initialized?"=w225, "TCP Listener"=w231) -> (w230:T4)
        n81 = call <vilib>:"Clear Errors.vi"("error in (no error)"=w224) -> ("error out"=w226:errorcluster)  [unwired: 5 in, 1 out]
        n82 = call <vilib>:"Add State(s) to Queue__JKI_lib_State_Machine.vi"("State(s) in Front (\"\")"=w228, "State(s) in (\"\")"=w242) -> ("States Out"=w241:string)  [unwired: 13 in]
      }
      frame "TCP: Listen" {
        # "TCP: Listen\n(Check for TCP connection until error or connection is made.)"
        n83 = Unbundle By Name(w248) -> ("Initialized?"=w244:bool, "TCP Listener"=w247:refnum<class "VISA TCP Listener.lvclass">)
        n84 = call-dynamic "Wait on Listener.vi"("error in (no error)"=w253, "timeout ms (5000)"=1000, "VISA TCP Listener in"=w247) -> ("error out"=w245:errorcluster, "Socket out"=w251:refnum<class "Socket.lvclass">)  [unwired: 6 in, 1 out]
        n85 = Select(t=TRUE, s=w245, f=w244) -> (s? t:f=w243:bool)
        n86 = Bundle By Name(cluster=w248, "Initialized?"=w243, "Socket"=w251) -> (w252:T4)
        n87 = case shown="Error 56" w245 {
          selector: w245 -> [w257 w260 w263]
          tunnel: [w257 w260 w262] -> w250
          tunnel: ["TCP: Close\nWebSocket: Initialize" "TCP: Initialize" "Macro: Run Process\nTCP: Listen"] -> w249
          frame No Error {
            # "Incoming connection - try to upgrade to WebSocket\nClose listener while connection is active."
          }
          frame Default {
            # "Unknown error - reset listener."
          }
          frame Error {
            # "Timeout - ignore"
            n88 = call <vilib>:"Clear Errors.vi"("error in (no error)"=w263) -> ("error out"=w262:errorcluster)  [unwired: 5 in, 1 out]
          }
        }
        n89 = call <vilib>:"Add State(s) to Queue__JKI_lib_State_Machine.vi"("State(s) in (\"\")"=w256, "State(s) at Back (\"\")"=w249) -> ("States Out"=w255:string)  [unwired: 13 in]
      }
      frame "TCP: Close" {
        # "TCP: Close\n(Close open TCP connection.)"
        n90 = Unbundle By Name(w269) -> ("TCP Listener"=w270:refnum<class "VISA TCP Listener.lvclass">)
        n91 = Bundle By Name(cluster=w269, "TCP Listener"=refnum<class "VISA TCP Listener.lvclass"> refnum) -> (w267:T4)
        n92 = call-dynamic "Close.vi"("error in (no error)"=w271, "VISA TCP Listener in"=w270) -> ("error out"=w266:errorcluster)  [unwired: 9 in]
        n93 = case shown="\"Ignore Errors\"" w264 {
          tunnel: w266 -> [w274 w276]
          tunnel: [w274 w275] -> w265
          frame Default {
          }
          frame "Ignore Errors" {
            n94 = call <vilib>:"Clear Errors.vi"("error in (no error)"=w276) -> ("error out"=w275:errorcluster)  [unwired: 5 in, 1 out]
          }
        }
        n95 = call <vilib>:"Add State(s) to Queue__JKI_lib_State_Machine.vi"("State(s) in (\"\")"=w273) -> ("States Out"=w272:string)  [unwired: 14 in]
      }
      frame "---------- WebSocket ----------" {
        # "Do not put any code in this frame.\n(It is a separator no-op. You can make a copy of this frame to create a new WebSocket frame)"
        n96 = call <vilib>:"Add State(s) to Queue__JKI_lib_State_Machine.vi"("State(s) in (\"\")"=w280) -> ("States Out"=w279:string)  [unwired: 14 in]
      }
      frame "WebSocket: Initialize" {
        # "WebSocket: Initialize\n(Try and upgrade to a WebSocket connection.)"
        n97 = Unbundle By Name(w289) -> ("Initialized?"=w281:bool, "Socket"=w292:refnum<class "Socket.lvclass">)
        n98 = call <vilib>:"New Server from Socket.vi"("error in (no error)"=w291, "Socket"=w292) -> ("error out"=w290:errorcluster, "WebSocket Server out"=w293:refnum<class "WebSocket Server.lvclass">)  [unwired: 8 in]
        n99 = call-dynamic "Handshake.vi"("error in (no error)"=w290, "WebSocket Connection in"=w293) -> ("error out"=w283:errorcluster, "WebSocket Connection out"=w288:refnum<class "WebSocket Server.lvclass">)  [unwired: 8 in]
        n100 = Bundle By Name(cluster=w289, "Initialized?"=TRUE, "WebSocket"=w288) -> (w286:T4)
        n101 = case shown="No Error" w283 {
          selector: w283 -> [w303 w306]
          tunnel: [w303 w307] -> w287
          tunnel: w286 -> [w302 w305]
          tunnel: [w300 w305] -> w284
          tunnel: [w299 "TCP: Initialize"] -> w285
          tunnel: w281 -> [w298 _]
          frame No Error {
            n102 = Bundle By Name(cluster=w302, "Websocket Connected?"=TRUE) -> (w300:T4)
            n103 = Select(t="Project: Sync Web UI", s=w298, f="Project: Initialize from Web UI") -> (s? t:f=w299:string)
          }
          frame Error {
            n104 = call <vilib>:"Clear Errors.vi"("error in (no error)"=w306) -> ("error out"=w307:errorcluster)  [unwired: 5 in, 1 out]
          }
        }
        n105 = call <vilib>:"Add State(s) to Queue__JKI_lib_State_Machine.vi"("State(s) in (\"\")"=w295, "State(s) at Back (\"\")"=w285) -> ("States Out"=w294:string)  [unwired: 13 in]
      }
      frame "WebSocket: Read" {
        # "WebSocket: Read\n(Check for incoming WebSocket data and process if available.)"
        n106 = Unbundle By Name(w312) -> ("WebSocket"=w314:refnum<class "WebSocket Server.lvclass">)
        n107 = call-dynamic "Read Text.vi"("error in (no error)"=w316, "timeout ms (5000)"=250, "WebSocket in"=w314) -> ("error out"=w315:errorcluster, "Data"=w308:string, "WebSocket out"=w313:refnum<class "WebSocket Server.lvclass">)  [unwired: 6 in]
        n108 = Bundle By Name(cluster=w312, "WebSocket"=w313, "JSON Data In"=w308) -> (w309:T4)
        n109 = case shown="No Error" w315 {
          selector: w315 -> [w321 w323 w327]
          tunnel: [w321 w322 w326] -> w311
          tunnel: ["Project: Process JSON" "WebSocket: Close" ""] -> w310
          frame No Error {
            # "Incoming Command - Process"
          }
          frame Default {
            # "Unknown error - Close Connection and Re-initialize"
            n110 = call <vilib>:"Clear Errors.vi"("error in (no error)"=w323) -> ("error out"=w322:errorcluster)  [unwired: 5 in, 1 out]
          }
          frame Error {
            # "Timeout - ignore"
            n111 = call <vilib>:"Clear Errors.vi"("error in (no error)"=w327) -> ("error out"=w326:errorcluster)  [unwired: 5 in, 1 out]
          }
        }
        n112 = call <vilib>:"Add State(s) to Queue__JKI_lib_State_Machine.vi"("State(s) in Front (\"\")"=w310, "State(s) in (\"\")"=w319) -> ("States Out"=w318:string)  [unwired: 13 in]
      }
      frame "WebSocket: Write" {
        # "WebSocket: Write\n(Write the data to be published over the WebSocket.)"
        n113 = Unbundle By Name(w338) -> ("WebSocket"=w336:refnum<class "WebSocket Server.lvclass">, "JSON Data Out"=w328:string)
        n114 = call-dynamic "Write Text.vi"("error in (no error)"=w333, "timeout ms (5000)"=1000, "String Data"=w328, "WebSocket in"=w336) -> ("error out"=w329:errorcluster, "WebSocket out"=w334:refnum<class "WebSocket Server.lvclass">)  [unwired: 6 in]
        n115 = Bundle By Name(cluster=w338, "WebSocket"=w334) -> (w337:T4)
        n116 = Select(t="WebSocket: Close", s=w329, f="") -> (s? t:f=w331:string)
        n117 = call <vilib>:"Clear Errors.vi"("error in (no error)"=w329) -> ("error out"=w330:errorcluster)  [unwired: 5 in, 1 out]
        n118 = call <vilib>:"Add State(s) to Queue__JKI_lib_State_Machine.vi"("State(s) in Front (\"\")"=w331, "State(s) in (\"\")"=w341) -> ("States Out"=w340:string)  [unwired: 13 in]
      }
      frame "WebSocket: Close" {
        # "Could occur based on when connection is closed."
        # "WebSocket: Close\n(Close open WebSocket connection and try to reconnect.)"
        n119 = Unbundle By Name(w350) -> ("WebSocket"=w351:refnum<class "WebSocket Server.lvclass">)
        n120 = Bundle By Name(cluster=w350, "WebSocket"=refnum<class "WebSocket Server.lvclass"> refnum, "Websocket Connected?"=FALSE) -> (w348:T4)
        n121 = call-dynamic "Close.vi"("error in (no error)"=w352, "timeout ms (5000)"=250, "WebSocket in"=w351) -> ("error out"=w347:errorcluster)  [unwired: 8 in]
        n122 = case shown="Default" w345 {
          tunnel: w347 -> [w357 w361]
          tunnel: [w356 w360] -> w346
          tunnel: ["TCP: Initialize" w359] -> w344
          tunnel: w343 -> [_ w359]
          frame Default {
            n123 = call <vilib>:"Clear Errors.vi"("error in (no error)"=w357, "specific error code to clear (0: all)"=66) -> ("error out"=w356:errorcluster)  [unwired: 4 in, 1 out]
          }
          frame "Ignore Errors" {
            n124 = call <vilib>:"Clear Errors.vi"("error in (no error)"=w361) -> ("error out"=w360:errorcluster)  [unwired: 5 in, 1 out]
          }
        }
        n125 = call <vilib>:"Add State(s) to Queue__JKI_lib_State_Machine.vi"("State(s) in (\"\")"=w344) -> ("States Out"=w354:string)  [unwired: 14 in]
      }
      frame "---------- Pi ----------" {
        # "Do not put any code in this frame.\n(It is a separator no-op. You can make a copy of this frame to create a new Pi frame)"
        n126 = call <vilib>:"Add State(s) to Queue__JKI_lib_State_Machine.vi"("State(s) in (\"\")"=w365) -> ("States Out"=w364:string)  [unwired: 14 in]
      }
      frame "Pi: Get Pi OS Time" {
        # "Pi: Get Pi OS Time\n(Get the current time of the Pi's primary OS.)"
        n127 = call <vilib>:"System Exec.vi"("error in (no error)"=w375, "command line"="ssh pi@localhost date") -> ("error out"=w372:errorcluster, "standard output"=w379:string)  [unwired: 6 in, 2 out]
        n128 = Match Pattern(string=w379, regular expression="\n") -> (before substring=w368:string)  [unwired: 1 in, 3 out]
        n129 = Format Into String(format string="Project: Determine Comms >> Pi OS Time,%s", w368) -> (resulting string=w366:string)  [unwired: 2 in, 1 out]
        n130 = Bundle By Name(cluster=cluster{"Command":string, "Pi OS Time":string} {"Command"="Pi OS Time", "Pi OS Time"=""}, "Pi OS Time"=w368) -> (w373:cluster{"Command":string, "Pi OS Time":string})
        n131 = call <vilib>:"Flatten To JSON String.vi"("error in (no error)"=w372, "Variant"=w373) -> ("error out"=w371:errorcluster, "JSON String"=w370:string)  [unwired: 8 in]
        n132 = Bundle By Name(cluster=w367, "Current Time.Pi OS"=w368, "JSON Data Out"=w370) -> (w376:T4)
        n133 = call <vilib>:"Add State(s) to Queue__JKI_lib_State_Machine.vi"("State(s) in Front (\"\")"=w366, "State(s) in (\"\")"=w381) -> ("States Out"=w380:string)  [unwired: 13 in]
      }
      frame "Pi: Get LabVIEW OS Time" {
        # "Pi: Get LabVIEW OS Time\n(Get the current time of the Pi OS LabVIEW is running on.)"
        n134 = call <vilib>:"System Exec.vi"("error in (no error)"=w392, "command line"="date") -> ("error out"=w388:errorcluster, "standard output"=w395:string)  [unwired: 6 in, 2 out]
        n135 = Match Pattern(string=w395, regular expression="\n") -> (before substring=w384:string)  [unwired: 1 in, 3 out]
        n136 = Format Into String(format string="Project: Determine Comms >> LV OS Time,%s", w384) -> (resulting string=w382:string)  [unwired: 2 in, 1 out]
        n137 = Bundle By Name(cluster=cluster{"Command":string, "LV OS Time":string} {"Command"="LV OS Time", "LV OS Time"=""}, "LV OS Time"=w384) -> (w389:cluster{"Command":string, "LV OS Time":string})
        n138 = call <vilib>:"Flatten To JSON String.vi"("error in (no error)"=w388, "Variant"=w389) -> ("error out"=w387:errorcluster, "JSON String"=w386:string)  [unwired: 8 in]
        n139 = Bundle By Name(cluster=w383, "Current Time.LabVIEW OS"=w384, "JSON Data Out"=w386) -> (w391:T4)
        n140 = call <vilib>:"Add State(s) to Queue__JKI_lib_State_Machine.vi"("State(s) in Front (\"\")"=w382, "State(s) in (\"\")"=w397) -> ("States Out"=w396:string)  [unwired: 13 in]
      }
      frame "Pi: Set Pi OS Timezone" {
        # "Pi: Set Pi OS Timezone\n(Command the Pi OS to set to the desired timezone.)"
        n141 = Unbundle By Name(w401) -> ("Current Timezone"=w400:string)
        n142 = Format Into String(format string="ssh pi@localhost sudo timedatectl set-timezone %s" ("command line"), w400) -> (resulting string=w403:string)  [unwired: 2 in, 1 out]
        n143 = call <vilib>:"System Exec.vi"("error in (no error)"=w399, "command line"=w403) -> ("error out"=w398:errorcluster)  [unwired: 6 in, 3 out]
        n144 = call <vilib>:"Add State(s) to Queue__JKI_lib_State_Machine.vi"("State(s) in (\"\")"=w405) -> ("States Out"=w404:string)  [unwired: 14 in]
      }
      frame "Pi: Set LabVIEW OS Timezone" {
        # "Pi: Set LabVIEW OS Timezone\n(Command the LabVIEW OS to set to the desired timezone.)"
        n145 = Unbundle By Name(w407) -> ("Current Timezone"=w406:string)
        n146 = Format Into String(format string="ln -sf /usr/share/zoneinfo/%s /etc/localtime" ("command line"), w406) -> (resulting string=w411:string)  [unwired: 2 in, 1 out]
        n147 = call <vilib>:"System Exec.vi"("error in (no error)"=w409, "command line"=w411) -> ("error out"=w408:errorcluster)  [unwired: 6 in, 3 out]
        n148 = call <vilib>:"Add State(s) to Queue__JKI_lib_State_Machine.vi"("State(s) in (\"\")"=w413) -> ("States Out"=w412:string)  [unwired: 14 in]
      }
      frame "Pi: Restart LabVIEW Service" {
        # "Pi: Restart LabVIEW Service\n(Command the LabVIEW Service to restart.)"
        n149 = call <vilib>:"System Exec.vi"("error in (no error)"=w416, "command line"="ssh pi@localhost sudo systemctl restart labview.service") -> ("error out"=w415:errorcluster)  [unwired: 6 in, 3 out]
        n150 = call <vilib>:"Add State(s) to Queue__JKI_lib_State_Machine.vi"("State(s) in (\"\")"=w419) -> ("States Out"=w418:string)  [unwired: 14 in]
      }
      frame "---------- Project ----------" {
        # "Do not put any code in this frame.\n(It is a separator no-op. You can make a copy of this frame to create a new Project frame)"
        n151 = call <vilib>:"Add State(s) to Queue__JKI_lib_State_Machine.vi"("State(s) in (\"\")"=w423) -> ("States Out"=w422:string)  [unwired: 14 in]
      }
      frame "Project: Get LabVIEW Time" {
        # "Project: Get LabVIEW Time\n(Get the current time from LabVIEW.)"
        n152 = Get Date/Time In Seconds() -> (seconds since 1Jan1904=w433:timestamp)
        n153 = Format Into String(format string="%<%c>T", w433) -> (resulting string=w426:string)  [unwired: 2 in, 1 out]
        n154 = Format Into String(format string="Project: Determine Comms >> LV Time,%s", w426) -> (resulting string=w424:string)  [unwired: 2 in, 1 out]
        n155 = Bundle By Name(cluster=cluster{"Command":string, "LV Time":string} {"Command"="LV Time", "LV Time"=""}, "LV Time"=w426) -> (w431:cluster{"Command":string, "LV Time":string})
        n156 = call <vilib>:"Flatten To JSON String.vi"("error in (no error)"=w429, "Variant"=w431) -> ("error out"=w428:errorcluster, "JSON String"=w430:string)  [unwired: 8 in]
        n157 = Bundle By Name(cluster=w425, "Current Time.LabVIEW"=w426, "JSON Data Out"=w430) -> (w435:T4)
        n158 = call <vilib>:"Add State(s) to Queue__JKI_lib_State_Machine.vi"("State(s) in Front (\"\")"=w424, "State(s) in (\"\")"=w437) -> ("States Out"=w436:string)  [unwired: 13 in]
      }
      frame "Project: Initialize from Web UI" {
        # "Project: Initialize from Web UI\n(Send the Command to get the current state of the Web UI.)"
        n159 = call <vilib>:"Flatten To JSON String.vi"("error in (no error)"=w442, "Variant"=cluster{"Command":string} {"Command"="Web UI State"}) -> ("error out"=w441:errorcluster, "JSON String"=w439:string)  [unwired: 8 in]
        n160 = Bundle By Name(cluster=w440, "JSON Data Out"=w439) -> (w438:T4)
        n161 = call <vilib>:"Add State(s) to Queue__JKI_lib_State_Machine.vi"("State(s) in Front (\"\")"="WebSocket: Write\nWebSocket: Read", "State(s) in (\"\")"=w446) -> ("States Out"=w445:string)  [unwired: 13 in]
      }
      frame "Project: Sync Web UI" {
        w451 = ""
        # "Project: Sync Web UI\n(Sync the current states to the Web UI.)"
        n162 = Unbundle By Name(w463) -> ("Websocket Connected?"=w462:bool, "SystemLink Booleans.Send SystemLink Messages?"=w452:bool, "SystemLink Booleans.Send SystemLink Tags?"=w455:bool, "SystemLink Booleans"=w450:T5)
        n163 = Unbundle By Name(w463) -> ("Enabled Booleans"=w473:T8, "Timezone Booleans"=w472:T7)
        n164 = Cluster To Array(cluster=w473) -> (array=w471:bool[])
        n165 = Cluster To Array(cluster=w472) -> (array=w470:bool[])
        n166 = call <userlib>:"Get Cluster Element Names__ogtk.vi"("Cluster"=w473) -> ("Element Names"=w468:string[])  [unwired: 9 in, 1 out]
        n167 = call <userlib>:"Get Cluster Element Names__ogtk.vi"("Cluster"=w472) -> ("Element Names"=w467:string[])  [unwired: 9 in, 1 out]
        n168 = local write "Sync"(FALSE) -> ()
        n169 = Build Array (concatenate)(w471, w470) -> (w469:bool[])
        n170 = Build Array (concatenate)(w468, w467) -> (w466:string[])
        n171 = for {
          tunnel: [w496] -> w457 mode=indexing
          tunnel: w469 -> [w493] mode=indexing
          tunnel: w466 -> [w494] mode=indexing
          shift-right: [w491] -> w464
          shift-left: "" -> [w489]
          n172 = Empty String/Path?(string/path=w489) -> (empty?=w492:bool)
          n173 = Format Into String(format string="SystemLink: Write Tag >> %s,%s", w494, w493) -> (resulting string=w487:string)  [unwired: 2 in, 1 out]
          n174 = Bundle By Name(cluster=cluster{"Name":string, "Value":bool} {"Name"="", "Value"=FALSE}, "Value"=w493, "Name"=w494) -> (w496:cluster{"Name":string, "Value":bool})
          n175 = Format Into String(format string="%s\n%s", w489, w487) -> (resulting string=w488:string)  [unwired: 2 in, 1 out]
          n176 = Select(t=w487, s=w492, f=w488) -> (s? t:f=w491:string)
        }
        n177 = Cluster To Array(cluster=w450) -> (array=w448:bool[])
        n178 = call <userlib>:"Get Cluster Element Names__ogtk.vi"("Cluster"=w450) -> ("Element Names"=w449:string[])  [unwired: 9 in, 1 out]
        n179 = for {
          tunnel: w449 -> [w485] mode=indexing
          tunnel: w448 -> [w484] mode=indexing
          tunnel: [w483] -> w447 mode=indexing
          n180 = Bundle By Name(cluster=cluster{"Name":string, "Value":bool} {"Name"="", "Value"=FALSE}, "Name"=w485, "Value"=w484) -> (w483:cluster{"Name":string, "Value":bool})
        }
        n181 = Build Array (concatenate)(w457, w447) -> (w456:cluster{"Name":string, "Value":bool}[])
        n182 = Bundle By Name(cluster=T1 {"Command"="Sync Web UI", "Controls"=[]}, "Controls"=w456) -> (w476:T1)
        n183 = Select(t="WebSocket: Write", s=w462, f=w451) -> (s? t:f=w459:string)
        n184 = Select(t="SystemLink: Write Message", s=w452, f=w451) -> (s? t:f=w453:string)
        n185 = Select(t=w464, s=w455, f=w451) -> (s? t:f=w458:string)
        n186 = call <vilib>:"Flatten To JSON String.vi"("error in (no error)"=w480, "Variant"=w476) -> ("error out"=w479:errorcluster, "JSON String"=w478:string)  [unwired: 8 in]
        n187 = call <vilib>:"Add State(s) to Queue__JKI_lib_State_Machine.vi"("State(s) in Front (\"\")"=w459, "State(s) in (\"\")"=w453, "State(s) at Back (\"\")"=w458) -> ("States Out"=w461:string)  [unwired: 12 in]
        n188 = Bundle By Name(cluster=w463, "JSON Data Out"=w478) -> (w477:T4)
        n189 = call <vilib>:"Add State(s) to Queue__JKI_lib_State_Machine.vi"("State(s) in Front (\"\")"=w461, "State(s) in (\"\")"=w482) -> ("States Out"=w481:string)  [unwired: 13 in]
      }
      frame "Project: Determine Comms" {
        w503 = ""
        # "Project: Determine Comms\n(Determine which communication methods are enabled and trigger those cases.)"
        n190 = Unbundle By Name(w499) -> ("Websocket Connected?"=w506:bool, "SystemLink Booleans.Send SystemLink Messages?"=w502:bool, "SystemLink Booleans.Send SystemLink Tags?"=w504:bool)
        n191 = Format Into String(format string="SystemLink: Write Tag >> %s", w500) -> (resulting string=w507:string)  [unwired: 2 in, 1 out]
        n192 = Select(t="WebSocket: Write", s=w506, f=w503) -> (s? t:f=w509:string)
        n193 = Select(t="SystemLink: Write Message", s=w502, f=w503) -> (s? t:f=w501:string)
        n194 = Select(t=w507, s=w504, f=w503) -> (s? t:f=w508:string)
        n195 = call <vilib>:"Add State(s) to Queue__JKI_lib_State_Machine.vi"("State(s) in Front (\"\")"=w509, "State(s) in (\"\")"=w501, "State(s) at Back (\"\")"=w508) -> ("States Out"=w498:string)  [unwired: 12 in]
        n196 = call <vilib>:"Add State(s) to Queue__JKI_lib_State_Machine.vi"("State(s) in Front (\"\")"=w498, "State(s) in (\"\")"=w514) -> ("States Out"=w513:string)  [unwired: 13 in]
      }
      frame "Project: Process JSON" {
        w525 = cluster{"Command":string} {"Command"=""}
        # "Project: Process JSON\n(Process the JSON data.)"
        n197 = Unbundle By Name(w522) -> ("JSON Data In"=w521:string)
        n198 = call <vilib>:"Unflatten From JSON String.vi"("Type and Defaults"=w525, "error in (no error)"=w524, "JSON String"=w521) -> ("error out"=w530:errorcluster, "Variant"=w526:variant)  [unwired: 7 in]
        n199 = Variant To Data(error in=w530, type=w525, Variant=w526) -> (data=w528:cluster{"Command":string}, error out=w529:errorcluster)
        n200 = Unbundle By Name(w528) -> ("Command"=w527:string)
        n201 = case shown="\"Sync Web UI\"" w527 {
          tunnel: ["" "Command: Timezone" "Command: Process Boolean" "Command: Process Boolean >> Private" "Command: Process Web UI State" "Project: Sync Web UI"] -> w517
          tunnel: w529 -> [w534 w536 w538 w540 w542 w544]
          tunnel: [w534 w536 w538 w540 w542 w544] -> w523
          frame Default {
            # "Unknown Command"
          }
          frame "Timezone" {
            # "Process Timezone Command"
          }
          frame "LV Enabled", "LV OS Enabled", "LV OS TZ Update", "LV TZ Update", "Pi OS Enabled", "Pi OS TZ Update" {
            # "Process a Boolean Command"
          }
          frame "Send SystemLink Messages?", "Send SystemLink Tags?" {
            # "Process a Private Boolean Command"
          }
          frame "Web UI State" {
            # "Process the Web UI State Command"
          }
          frame "Sync Web UI" {
            # "Process the Sync Web UI Command"
          }
        }
        n202 = Empty String/Path?(string/path=w516) -> (empty?=w519:bool)
        n203 = Format Into String(format string="%s >> %s", w517, w516) -> (resulting string=w515:string)  [unwired: 2 in, 1 out]
        n204 = Select(t=w517, s=w519, f=w515) -> (s? t:f=w518:string)
        n205 = call <vilib>:"Add State(s) to Queue__JKI_lib_State_Machine.vi"("State(s) in Front (\"\")"=w518, "State(s) in (\"\")"=w532) -> ("States Out"=w531:string)  [unwired: 13 in]
      }
      frame "---------- Command ----------" {
        # "Do not put any code in this frame.\n(It is a separator no-op. You can make a copy of this frame to create a new Command frame)"
        n206 = call <vilib>:"Add State(s) to Queue__JKI_lib_State_Machine.vi"("State(s) in (\"\")"=w548) -> ("States Out"=w547:string)  [unwired: 14 in]
      }
      frame "Command: Timezone" {
        w555 = cluster{"Timezone":string} {"Timezone"=""}
        # "If the Timezone change is coming in from the Web Interface we \nneed to update here otherwise UI: Process Timezone will overwrite it."
        # "Command: Timezone\n(If the Timezone has changed call the Set Timezone Macro to perform update. )"
        n207 = Unbundle By Name(w553) -> ("Current Timezone"=w550:string, "JSON Data In"=w556:string)
        n208 = call <vilib>:"Unflatten From JSON String.vi"("Type and Defaults"=w555, "error in (no error)"=w559, "JSON String"=w556) -> ("error out"=w558:errorcluster, "Variant"=w557:variant)  [unwired: 7 in]
        n209 = Variant To Data(error in=w558, type=w555, Variant=w557) -> (data=w563:cluster{"Timezone":string}, error out=w560:errorcluster)
        n210 = Unbundle By Name(w563) -> ("Timezone"=w549:string)
        n211 = Bundle By Name(cluster=w553, "Current Timezone"=w549) -> (w552:T4)
        n212 = local write "Timezone"(w549) -> ()
        n213 = Equal?(x=w549, y=w550) -> (x = y?=w562:bool)
        n214 = Select(t="", s=w562, f="Macro: Set Timezone") -> (s? t:f=w554:string)
        n215 = call <vilib>:"Add State(s) to Queue__JKI_lib_State_Machine.vi"("State(s) in Front (\"\")"=w554, "State(s) in (\"\")"=w565) -> ("States Out"=w564:string)  [unwired: 13 in]
      }
      frame "Command: Process Boolean" {
        w570 = "SystemLink Message"
        w567 = ""
        w592 = cluster{"Command":string, "Enabled?":bool} {"Command"="", "Enabled?"=FALSE}
        # "Command: Process Boolean\n(Set the appropriate boolean control based on the command.)"
        n216 = Unbundle By Name(w575) -> ("JSON Data In"=w574:string)
        n217 = call <vilib>:"Unflatten From JSON String.vi"("Type and Defaults"=w592, "error in (no error)"=w595, "JSON String"=w574) -> ("error out"=w594:errorcluster, "Variant"=w593:variant)  [unwired: 7 in]
        n218 = Bundle By Name(cluster=w575, "JSON Data Out"=w574) -> (w573:T4)
        n219 = Variant To Data(error in=w594, type=w592, Variant=w593) -> (data=w596:cluster{"Command":string, "Enabled?":bool}, error out=w591:errorcluster)
        n220 = Equal?(x=w571, y=w570) -> (x = y?=w569:bool)
        n221 = Not Equal?(x=w571, y="Private") -> (x != y?=w581:bool)
        n222 = Not Equal?(x=w571, y=w570) -> (x != y?=w572:bool)
        n223 = Unbundle By Name(w596) -> ("Command"=w589:string, "Enabled?"=w588:bool)
        n224 = Unbundle By Name(w573) -> ("SystemLink Booleans.Send SystemLink Messages?"=w580:bool, "SystemLink Booleans.Send SystemLink Tags?"=w583:bool)
        n225 = case shown="\"Send SystemLink Messages?\"" w589 {
          selector: w589 -> [w600 _ _ _ _ _ _ _ _]
          tunnel: w588 -> [_ w608 w610 w612 w614 w616 w618 w620 w622]
          tunnel: w591 -> [_ w609 w611 w613 w615 w617 w619 w621 w623]
          tunnel: [w599 w609 w611 w613 w615 w617 w619 w621 w623] -> w582
          frame Default {
            # "Unknown Boolean Command"
            n226 = xnode "Error Ring"("parameter 0"=w600) -> ("error out"=w599:errorcluster)
          }
          frame "LV Enabled" {
            # "Update LV Enable Boolean"
            n227 = local write "LV Enabled"(w608) -> ()
          }
          frame "LV OS Enabled" {
            # "Update LV OS Enable Boolean"
            n228 = local write "LV OS Enabled"(w610) -> ()
          }
          frame "Pi OS Enabled" {
            # "Update Pi OS Enable Boolean"
            n229 = local write "Pi OS Enabled"(w612) -> ()
          }
          frame "LV TZ Update" {
            # "Update LV TZ Update Boolean"
            n230 = local write "LV TZ Update"(w614) -> ()
          }
          frame "LV OS TZ Update" {
            # "Update LV OS TZ Update Boolean"
            n231 = local write "LV OS TZ Update"(w616) -> ()
          }
          frame "Pi OS TZ Update" {
            # "Update Pi OS TZ Update Boolean"
            n232 = local write "Pi OS TZ Update"(w618) -> ()
          }
          frame "Send SystemLink Tags?" {
            # "Update Send SystemLink Tags? Boolean"
            n233 = local write "Send SystemLink Tags?"(w620) -> ()
          }
          frame "Send SystemLink Messages?" {
            # "Update Send SystemLink Messages? Boolean"
            n234 = local write "Send SystemLink Messages?"(w622) -> ()
          }
        }
        n235 = Format Into String(format string="SystemLink: Write Tag >> %s,%s", w589, w588) -> (resulting string=w586:string)  [unwired: 2 in, 1 out]
        n236 = Compound Arithmetic op=AND(w581, w583, invert w582) -> (w587:bool)
        n237 = Compound Arithmetic op=AND(w572, w581, w580, invert w582) -> (w579:bool)
        n238 = Select(t="WebSocket: Write", s=w569, f=w567) -> (s? t:f=w566:string)
        n239 = Select(t="SystemLink: Write Message", s=w579, f=w567) -> (s? t:f=w578:string)
        n240 = Select(t=w586, s=w587, f=w567) -> (s? t:f=w584:string)
        n241 = call <vilib>:"Add State(s) to Queue__JKI_lib_State_Machine.vi"("State(s) in Front (\"\")"=w566, "State(s) in (\"\")"=w578, "State(s) at Back (\"\")"=w584) -> ("States Out"=w577:string)  [unwired: 12 in]
        n242 = call <vilib>:"Add State(s) to Queue__JKI_lib_State_Machine.vi"("State(s) in Front (\"\")"=w577, "State(s) in (\"\")"=w598) -> ("States Out"=w597:string)  [unwired: 13 in]
      }
      frame "Command: Process Web UI State" {
        w629 = T1 {"Command"="", "Controls"=[]}
        # "Command: Process Web UI State\n(Set the appropriate control to the state on the Web UI.)"
        n243 = Unbundle By Name(w628) -> ("JSON Data In"=w630:string)
        n244 = call <vilib>:"Unflatten From JSON String.vi"("Type and Defaults"=w629, "error in (no error)"=w633, "JSON String"=w630) -> ("error out"=w632:errorcluster, "Variant"=w631:variant)  [unwired: 7 in]
        n245 = Variant To Data(error in=w632, type=w629, Variant=w631) -> (data=w634:T1, error out=w626:errorcluster)
        n246 = Unbundle By Name(w634) -> ("Controls"=w624:cluster{"Name":string, "Value":bool}[])
        n247 = for {
          shift-right: [w640] -> w625
          shift-left: w626 -> [w641]
          tunnel: w624 -> [w639] mode=indexing
          # "For each control received."
          n248 = Unbundle By Name(w639) -> ("Name"=w638:string, "Value"=w637:bool)
          n249 = case shown="\"Send SystemLink Messages?\"" w638 {
            selector: w638 -> [w643 _ _ _ _ _ _ _ _]
            tunnel: w637 -> [_ w651 w653 w655 w657 w659 w661 w664 w665]
            tunnel: w641 -> [_ w652 w654 w656 w658 w660 w662 w663 w666]
            tunnel: [w642 w652 w654 w656 w658 w660 w662 w663 w666] -> w640
            frame Default {
              # "Unknown Boolean Command"
              n250 = xnode "Error Ring"("parameter 0"=w643) -> ("error out"=w642:errorcluster)
            }
            frame "LV Enabled" {
              # "Update LV Enable Boolean"
              n251 = local write "LV Enabled"(w651) -> ()
            }
            frame "LV OS Enabled" {
              # "Update LV OS Enable Boolean"
              n252 = local write "LV OS Enabled"(w653) -> ()
            }
            frame "Pi OS Enabled" {
              # "Update Pi OS Enable Boolean"
              n253 = local write "Pi OS Enabled"(w655) -> ()
            }
            frame "LV TZ Update" {
              # "Update LV TZ Update Boolean"
              n254 = local write "LV TZ Update"(w657) -> ()
            }
            frame "LV OS TZ Update" {
              # "Update LV OS TZ Update Boolean"
              n255 = local write "LV OS TZ Update"(w659) -> ()
            }
            frame "Pi OS TZ Update" {
              # "Update Pi OS TZ Update Boolean"
              n256 = local write "Pi OS TZ Update"(w661) -> ()
            }
            frame "Send SystemLink Tags?" {
              # "Update Send SystemLink Tags? Boolean"
              n257 = local write "Send SystemLink Tags?"(w664) -> ()
            }
            frame "Send SystemLink Messages?" {
              # "Update Send SystemLink Messages? Boolean"
              n258 = local write "Send SystemLink Messages?"(w665) -> ()
            }
          }
        }
        n259 = call <vilib>:"Add State(s) to Queue__JKI_lib_State_Machine.vi"("State(s) in Front (\"\")"="UI: Update Booleans", "State(s) in (\"\")"=w636) -> ("States Out"=w635:string)  [unwired: 13 in]
      }
      frame "---------- SystemLink ----------" {
        # "Do not put any code in this frame.\n(It is a separator no-op. You can make a copy of this frame to create a new Command frame)"
        n260 = call <vilib>:"Add State(s) to Queue__JKI_lib_State_Machine.vi"("State(s) in (\"\")"=w670) -> ("States Out"=w669:string)  [unwired: 14 in]
      }
      frame "SystemLink: Initialize" {
        # "SystemLink: Initialize\n(Configure the SystemLink Cloud connection and all the tags.)"
        n261 = call-poly <vilib>:"Open Configuration.vi"("error in (no error)"=w681, "api key"="Z11BYcjG7Q5ZNKbdVo3Ssxbzi7Re2rE2teXJZWmEuD", "server url"="https://api.systemlinkcloud.com") -> ("error out"=w676:errorcluster, "configuration"=w677:refnum<class "NI Skyline Configuration HTTP.lvclass">)  [unwired: 7 in]
        n262 = for {
          tunnel: w676 -> [w697]
          tunnel: [w696] -> w679 mode=indexing
          tunnel: [w693] -> w678 mode=indexing
          tunnel: cluster{"Path":string, "Data Type":T2}[] [{"Path"="LV Time", "Data Type"=enum."String"}, {"Path"="LV OS Time", "Data Type"=enum."String"}, {"Path"="Pi OS Time", "Data Type"=enum."String"}, {"Path"="LV Enabled", "Data Type"=enum."Boolean"}, {"Path"="LV OS Enabled", "Data Type"=enum."Boolean"}, {"Path"="Pi OS Enabled", "Data Type"=enum."Boolean"}, {"Path"="LV TZ Update", "Data Type"=enum."Boolean"}, {"Path"="LV OS TZ Update", "Data Type"=enum."Boolean"}, {"Path"="Pi OS TZ Update", "Data Type"=enum."Boolean"}] -> [w692] mode=indexing
          tunnel: w677 -> [w689]
          # "For each tag."
          n263 = Unbundle By Name(w692) -> ("Path"=w691:string, "Data Type"=w690:T2)
          n264 = call-poly <vilib>:"Open Tag 2.vi"("configuration"=w689, "error in (no error)"=w697, "Data Type"=w690, "path"=w691) -> ("error out"=w696:errorcluster, "tag"=w694:refnum<class "NI Skyline Tag.lvclass">)  [unwired: 6 in]
          n265 = Bundle By Name(cluster=T3 {"Name"="", "Reference"=refnum} ("Tag Info"), "Name"=w691, "Reference"=w694) -> (w693:T3)
        }
        n266 = call-poly <vilib>:"Open 2.vi"("configuration"=w677, "error in (no error)"=w676) -> ("error out"=w672:errorcluster, "message session"=w675:refnum<class "NI Skyline Message HTTP.lvclass">)  [unwired: 8 in]
        n267 = call-dynamic "Subscribe.vi"("error in (no error)"=w672, "topic"="CloudTest.Message.In", "message session in"=w675) -> ("error out"=w673:errorcluster, "message session out"=w674:refnum<class "NI Skyline Message HTTP.lvclass">)  [unwired: 7 in]
        n268 = Merge Errors(w673, w679) -> (w682:errorcluster)
        n269 = Bundle By Name(cluster=w684, "SystemLink Message Session"=w674, "SystemLink Tag Info"=w678) -> (w683:T4)
        n270 = call <vilib>:"Add State(s) to Queue__JKI_lib_State_Machine.vi"("State(s) in (\"\")"=w688) -> ("States Out"=w687:string)  [unwired: 14 in]
      }
      frame "SystemLink: Read Message" {
        # "SystemLink: Read Message\n(Check for incoming SystemLink message and process if available.)"
        n271 = Unbundle By Name(w708) -> ("SystemLink Message Session"=w706:refnum<class "NI Skyline Message HTTP.lvclass">)
        n272 = call-dynamic "Read.vi"("error in (no error)"=w707, "sync message session in"=w706) -> ("error out"=w704:errorcluster, "message"=w703:string, "sync message session out"=w705:refnum<class "NI Skyline Message HTTP.lvclass">, "dequeue status"=w701:bool)  [unwired: 5 in, 1 out]
        n273 = Bundle By Name(cluster=w708, "SystemLink Message Session"=w705, "JSON Data In"=w703) -> (w702:T4)
        n274 = Select(t="Project: Process JSON >> SystemLink Message", s=w701, f="") -> (s? t:f=w698:string)
        n275 = call <vilib>:"Add State(s) to Queue__JKI_lib_State_Machine.vi"("State(s) in Front (\"\")"=w698, "State(s) in (\"\")"=w710) -> ("States Out"=w709:string)  [unwired: 13 in]
      }
      frame "SystemLink: Write Tag" {
        # "SystemLink: Write Tag\n(Write the tag data to be published to SystemLink.)"
        n276 = Unbundle By Name(w715) -> ("SystemLink Tag Info"=w716:T6)
        n277 = Spreadsheet String To Array(delimiter (Tab)=",", format string="%s", spreadsheet string=w726, array type (2D Dbl)="") -> (array=w723:string[][])
        n278 = Index Array(array=w723, index (row)=0 ("disabled index (col)")) -> (element=w722:string[])  [unwired: 1 in]
        n279 = Index Array(array=w722) -> (element #1=w720:string, element #2=w721:string)  [unwired: 2 in]
        n280 = for {
          tunnel: w716 -> [w779] mode=indexing
          tunnel: w720 -> [w777]
          tunnel: [w776] -> w718
          tunnel: [w775] -> w719
          tunnel: [w774] -> w717
          i -> [w774]
          stop <- w775 stop-if-true
          # "For each tag."
          n281 = Unbundle By Name(w779) -> ("Reference"=w776:refnum<class "NI Skyline Tag.lvclass">, "Name"=w778:string)
          n282 = Equal?(x=w778, y=w777) -> (x = y?=w775:bool)
        }
        n283 = case shown="True" w719 {
          tunnel: w728 -> [_ w751]
          tunnel: [w732 w750] -> w727
          tunnel: w721 -> [_ w749]
          tunnel: w720 -> [w733 w748]
          tunnel: w718 -> [_ w747]
          tunnel: w717 -> [_ w744]
          tunnel: w716 -> [w731 w743]
          tunnel: [w731 w742] -> w713
          frame False {
            # "Tag not configured in SystemLink: Initialize case."
            n284 = xnode "Error Ring"("parameter 0"=w733) -> ("error out"=w732:errorcluster)
          }
          frame True {
            # "Tag is configured in SystemLink: Initialize case."
            n285 = case shown="\"LV Enabled\", \"LV OS Enabled\", \"LV OS TZ Update\", \"LV TZ Update\", \"Pi OS Enabled\", \"Pi OS TZ Update\"" w748 {
              selector: w748 -> [w753 _ _]
              tunnel: w751 -> [_ w766 w773]
              tunnel: [w754 w765 w772] -> w750
              tunnel: w749 -> [_ w764 w769]
              tunnel: w747 -> [w752 w763 w771]
              tunnel: [w752 w762 w770] -> w741
              frame Default {
                n286 = xnode "Error Ring"("parameter 0"=w753) -> ("error out"=w754:errorcluster)
              }
              frame "LV OS Time", "LV Time", "Pi OS Time" {
                # "String Tags"
                n287 = call-poly <vilib>:"Write Tag.vi"("error in (no error)"=w766, "value"=w764, "tag in"=w763) -> ("error out"=w765:errorcluster, "tag out"=w762:refnum<class "NI Skyline Tag.lvclass">)  [unwired: 7 in]
              }
              frame "LV Enabled", "LV OS Enabled", "LV OS TZ Update", "LV TZ Update", "Pi OS Enabled", "Pi OS TZ Update" {
                # "String Tags"
                n288 = Equal?(x=w769, y="TRUE") -> (x = y?=w768:bool)
                n289 = call-poly <vilib>:"Write Tag.vi"("error in (no error)"=w773, "value"=w768, "tag in"=w771) -> ("error out"=w772:errorcluster, "tag out"=w770:refnum<class "NI Skyline Tag.lvclass">)  [unwired: 7 in]
              }
            }
            n290 = Index Array(array=w743, index=w744) -> (element=w745:T3)
            n291 = Bundle By Name(cluster=w745, "Reference"=w741) -> (w746:T3)
            n292 = Replace Array Subset(array=w743, new element=w746, index=w744) -> (w742:T6)
          }
        }
        n293 = Bundle By Name(cluster=w715, "SystemLink Tag Info"=w713) -> (w714:T4)
        n294 = call <vilib>:"Add State(s) to Queue__JKI_lib_State_Machine.vi"("State(s) in (\"\")"=w730) -> ("States Out"=w729:string)  [unwired: 14 in]
      }
      frame "SystemLink: Write Message" {
        # "SystemLink: Write Message\n(Write the message data to be published to SystemLink.)"
        n295 = Unbundle By Name(w783) -> ("SystemLink Message Session"=w786:refnum<class "NI Skyline Message HTTP.lvclass">, "JSON Data Out"=w780:string)
        n296 = call-dynamic "Publish.vi"("error in (no error)"=w785, "message"=w780, "topic"="CloudTest.Message.Out", "message session in"=w786) -> ("error out"=w784:errorcluster, "message session out"=w782:refnum<class "NI Skyline Message HTTP.lvclass">)  [unwired: 6 in]
        n297 = Bundle By Name(cluster=w783, "SystemLink Message Session"=w782) -> (w781:T4)
        n298 = call <vilib>:"Add State(s) to Queue__JKI_lib_State_Machine.vi"("State(s) in (\"\")"=w789) -> ("States Out"=w788:string)  [unwired: 14 in]
      }
      frame "SystemLink: Close" {
        # "SystemLink: Close\n(Cleanup SystemLink references.)"
        n299 = Unbundle By Name(w791) -> ("SystemLink Tag Info"=w790:T6)
        n300 = for {
          tunnel: w794 -> [w800]
          tunnel: [w799] -> w793 mode=indexing
          tunnel: w790 -> [w798] mode=indexing
          # "For each tag."
          n301 = Unbundle By Name(w798) -> ("Reference"=w797:refnum<class "NI Skyline Tag.lvclass">)
          n302 = call-poly <vilib>:"Close Tag.vi"("error in (no error)"=w800, "tag"=w797) -> ("error out"=w799:errorcluster)  [unwired: 9 in]
        }
        n303 = Merge Errors(w793) -> (w792:errorcluster)
        n304 = call <vilib>:"Add State(s) to Queue__JKI_lib_State_Machine.vi"("State(s) in (\"\")"=w796) -> ("States Out"=w795:string)  [unwired: 14 in]
      }
    }
  }
